vi "Measurement.vi"(0 "Position":T3(array[cluster]) {"Z" format="%.1f"; "Y" format="%.1f"; "X" format="%.1f"}, 1 "setup":T4=enum."Show Setup", 2 "Post Process":T2, 4 "File":T5, 5 "Results file":path, 7 "Raw data file":path, 11 "Setup filename":string) -> (14 "2nd plot":cluster{"X array":dbl[], "Y array":dbl[]}[](graph), 19 "Status Out":T1)   [LabVIEW 2015]
uses:
  Anemometry Sub Vis/Controls/Save_Data.ctl
  Anemometry Sub Vis/Controls/Setup.ctl
  Anemometry Sub Vis/Controls/Graph_Type.ctl
  Anemometry Sub Vis/Controls/Post_Process.ctl
  Anemometry Sub Vis/Gen Trav/Multi_Run_Status.ctl
  Anemometry Sub Vis/Controls/Inst_type.ctl
  ADAM Client/Sub VIs/ADAM Controls/Traverse_Level_State.ctl
  Anemometry Sub Vis/File/Setup_Filetype.ctl
  Anemometry Sub Vis/Globals/Meas_global.vi
  Anemometry Sub Vis/Globals/Trav_pos_global.vi
  Anemometry Sub Vis/Globals/Plug_in_data_global.vi
  Anemometry Sub Vis/Globals/Dynamic_call_global.ph.vi
  Anemometry Sub Vis/Globals/Preference_global.vi
  Anemometry Sub Vis/Globals/Constants_global.vi
  Anemometry Sub Vis/Globals/Extra_Commands_Global.vi
  Anemometry Sub Vis/Globals/LDA_meas_global_2.vi
  Anemometry Sub Vis/Globals/LDA_meas_global_1.vi
  Anemometry Sub Vis/Acquisition/PWA/PWAtasksGLOBAL.vi
  Anemometry Sub Vis/Acquisition/Data_Translation/DataTranslation_global.vi
  Anemometry Sub Vis/Globals/Gas_management_global.vi
panel:
  in  "PP next block":bool
  out "Pause message":string
  out "Statistics":string[][](table)
  out "Actual Sampling freq":dbl=100.0 format="%.1f"
  in  "Desired Sampling freq (Hz)":dbl=100.0 format="%.1f"
  out "Current Block No":i32=5 caption="Current Block"
  in  "Pause":bool
  in  "No of Blocks":i32=5
  in  "stop":bool
  in  "No of samples":i32=1000 min=0 step=1
  in  "Tab Control":T6(tab)
  in  "Second Graph":T8={"Plot 1"=2, "Plot 2"=1, "Save graph"=0, "Plot Type"=enum."Vel histogram"} {"Save graph" items=["Do not save plot", "Save plot"]; "Plot 2" items=["Nothing", "V"]; "Plot 1" items=["Nothing", "V"]}
  in  "First Graph":T8={"Plot 1"=1, "Plot 2"=2, "Save graph"=0, "Plot Type"=enum."Velocity trace"} {"Save graph" items=["Do not save plot", "Save plot"]; "Plot 2" items=["Nothing", "V"]; "Plot 1" items=["Nothing", "V"]}
  out "First plot":cluster{"X array":dbl[], "Y array":dbl[]}[](graph)
  in  "Comments":string
  out "uv":dbl[][](graph)=[[-0.041806189081711534, -0.046435429052714985, -0.04035660097427599, -0.042187605126076694, -0.042052555599004206]]
  out "u^4":dbl[][](graph)
  out "u^3":dbl[][](graph)
  out "u^2":dbl[][](graph)=[[0.09743628875280319, 0.10575821456272283, 0.10126262927293661, 0.09890442087602569, 0.1022948212436432]]
  out "U":dbl[][](graph)=[[0.8295029456391334, 0.8915896983798417, 0.8415763502225625, 0.8394746126219594, 0.8466062785395404]]
  in  "Block average display control":cluster{"Name":string, "Include":bool}[](array[cluster])=[{"Name"="FF (C)", "Include"=FALSE}]
  in  "No of bins in histogram":i32=100
  out "Measurement time (min)":dbl=6.0 format="%.2f"
  in  "Correlate?":T9(ring)
  out "Diagnostic info":string[][](table)
  out "Array U":dbl[][](array[numeric]) format="%.2e"
  out "Array u^2":dbl[][](array[numeric]) format="%.2e"
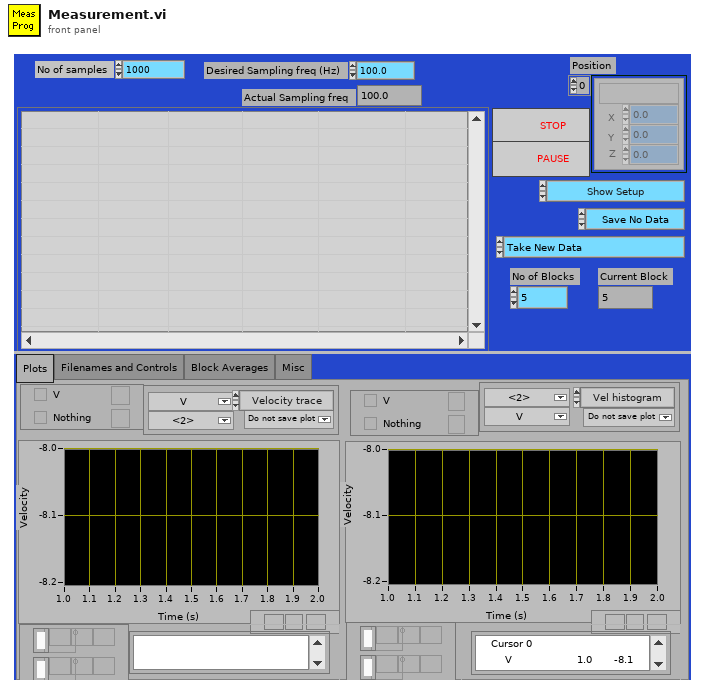
[diagram p1: front panel]
types:
  T1 = typedef "Multi_Run_Status.ctl" = enum16{"Continue", "Jump to Next Point", "Jump to Next Row", "Jump To Fall Back", "Terminate Run"}
  T2 = typedef "Post_Process.ctl" = enum16{"Take New Data", "Post Process Raw Data File"}
  T3 = cluster{"Name":string, "X":dbl, "Y":dbl, "Z":dbl}[]
  T4 = typedef "Setup.ctl" = enum16{"Run Program", "Show Setup", "Save Current Setup", "Setup Front Panel"}
  T5 = typedef "Save_Data.ctl" = enum16{"Save No Data", "Save Data"}
  T6 = enum32{"Plots", "Filenames and Controls", "Block Averages", "Misc"}
  T7 = typedef "Graph_Type.ctl" = enum16{"Show no graph", "Voltage trace", "Velocity trace", "Vel histogram", "Spectrum", "f.E(f) v Log f", "Auto-Corr"}
  T8 = cluster{"Plot 1":u16, "Plot 2":u16, "Save graph":u16, "Plot Type":T7}
  T9 = enum16{"Cross correlation off", "Show correlation panel", "Correlate without activating panel"}
  T10 = enum32{"Bad", "Idle", "Run top level", "Running"}
  T11 = cluster{"Name":string, "X":dbl, "Y":dbl, "Z":dbl}
  T12 = enum16{"Velocity", "Transit time", "Arrival time"}
  T13 = enum16{"Save no data", "Save data in new files", "Save data in existing files"}
  T14 = typedef "Inst_type.ctl" = enum16{"Propeller anemometer", "Raw voltage", "Pressure Transducer", "Pitot-static tube", "Preston tube", "Hot wire", "Cross wire 1", "Cross wire 2", "Generic Linear", "Generic Polynomial", "Generic BackPoly", "Fast FID", "Thermocouple", "Cold wire", "Pulsed Wire", "LDA Vel", "LDA Tran time", "LDA Arr time", "Microphone"}
  T15 = enum16{"Zero or one", "One", "Zero or more", "One or more"}
  T16 = cluster{"Weighting":dbl[], "Time (ms)":dbl[], "Voltage":dbl[], "Eng Values":dbl[]}
  T17 = typedef "Traverse_Level_State.ctl" = enum16{"Running", "Complete"}
  T18 = typedef "Setup_Filetype.ctl" = enum16{"Measurement Setups", "Calibration Setups", "General", "Results File Plotter Setups", "Speed Calib Tweaks"}
  T19 = typedef "Traverse_cluster.ctl" = cluster{"Start X":sgl, "Start Y":sgl, "Start Z":sgl, "End X":sgl, "End Y":sgl, "End Z":sgl, "No. of pts.":i32, "Spacing":T20, "Filename":path, "Tunnel Speed":dbl, "Averaging time (min)":dbl, "Extra Commands":string, "Carrier_1 Q (l/min)":dbl, "Carrier_2 Q (l/min)":dbl, "Trace Gas Concentration (%)":dbl, "Specific Arguments":string, "Comments":string, "Row No":i32, "Row Type Selector":T21, "Completion time":string, "Row Duration (mins)":dbl, "No. of Valid pts.":i32, "Meas Setup File":string}
  T20 = typedef "Spacing.ctl" = enum16{"Linear", "Log", "Gauss", "Specified", "N/A"}
  T21 = typedef "Multi_run_mode.ctl" = enum16{"Move Traverse Only", "Set Tunnel Speed Only", "Set Source Only", "Set Measurement Conditions", "Single Measurement", "Vertical Profile", "Lateral Profile", "Longitudinal Profile", "Explore Volume", "Multi-Axis Profile", "Auto Calibrate", "Meas Fast FID Bkgnd", "Check Beam Power", "Scanning Valve Measurement", "Run VI Named:", "Set ADAM Ch", "Wait (minutes)", "Send Message", "Synchronize With:", "Fall Back to this Row", "Turn Off Row Repeating", "Blank Row", "Traverse 3D Volume"}
  T22 = typedef "Analysis_info_cluster.ctl" = cluster{"Colour":u32, "Inst type":T14, "Inst name":string, "Symbol":string, "Code name":string, "Extra Info":string, "Inst Array":T23, "Extra Titles":string[], "Extra Values":string[], "U":dbl, "u^2":dbl, "u^3":dbl, "u^4":dbl, "Skew_u":dbl, "Kurt_u":dbl, "Sd Error in Mean":dbl, "% u'/U":dbl, "X":dbl, "Y":dbl, "Z":dbl, "Timescale integral to 25%":dbl, "Sd Error in Variance":dbl, "Calib File":path, "Calib Constants":dbl[], "Output Position":bool, "Full Stats":bool, "Av Sampling Rate":dbl, "Av No of Samples":dbl, "Total Meas Time (s)":dbl, "ADAM Ch Name":string}
  T23 = typedef "Instrument_Array.ctl" = enum16{"PWA", "LDA", "Analogue"}
  T24 = typedef "LDA_Setup.ctl" = cluster{"dimensions":enum16{"1D", "2D"}, "Analogue Freq Multiplier":dbl}
  T25 = enum16{"Velocity", "Transit time", "Arrival time"}[]
  T26 = typedef "BSA_Type.ctl" = enum16{"57N11", "BSA F60"}
  T27 = typedef "BSA_info_Cluster.ctl" = cluster{"GPIB Address":string, "No of Check Bytes":i32, "Extra Info":string, "COLOUR":u32, "Wavelength (nm)":dbl}
  T28 = typedef "Ch_and_Spans.ctl" = cluster{"high limit (10V)":sgl, "low limit (-10V)":sgl, "Ch No":i16, "Var name":string, "Use Latest Calib":bool}
  T29 = cluster{"Weighting":dbl[], "Time (ms)":dbl[], "Voltage":dbl[], "Eng Values":dbl[]}[]
  T30 = cluster{"Insts for plotting[0]":u16, "Insts for plotting[1]":u16}
  T31 = typedef "PWA_Data.ctl" = enum16{"No PWA Data", "One Ch PWA"}
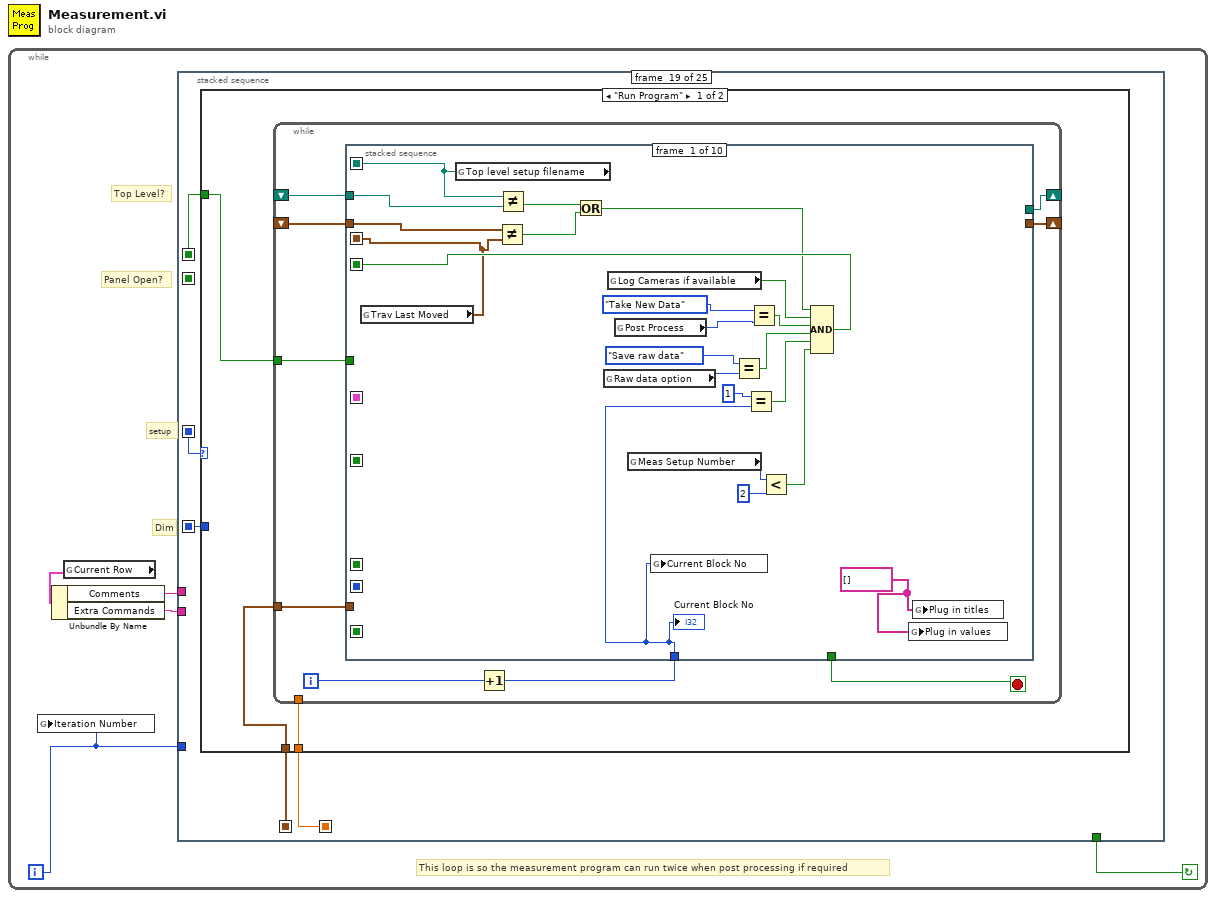
[diagram p0: block diagram]
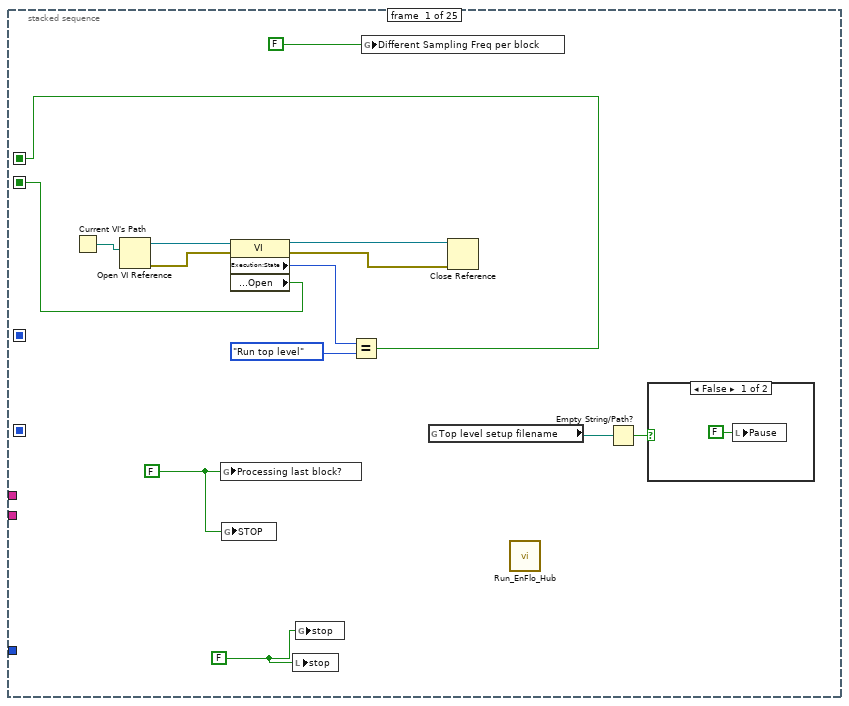
[diagram p2: hidden frame]
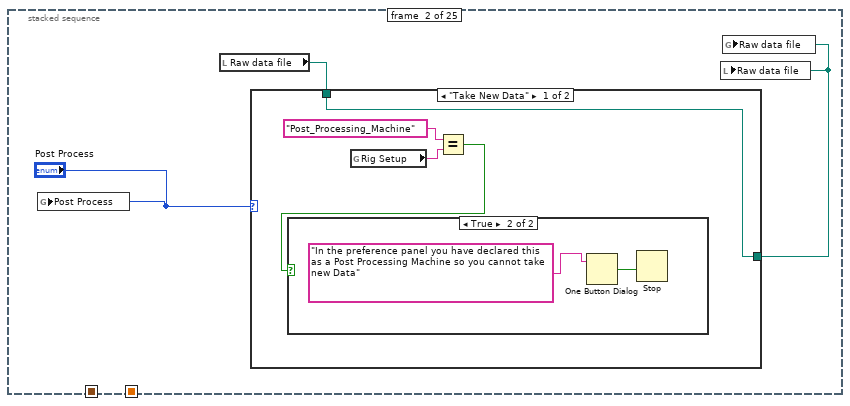
[diagram p4: hidden frame]
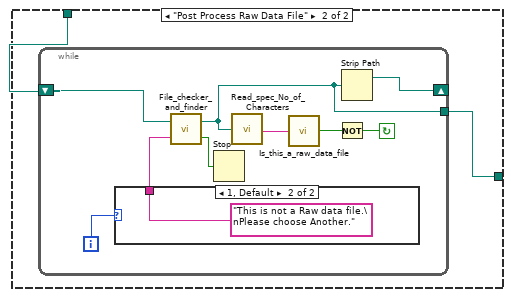
[diagram p6: hidden frame]
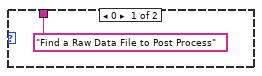
[diagram p7: hidden frame]
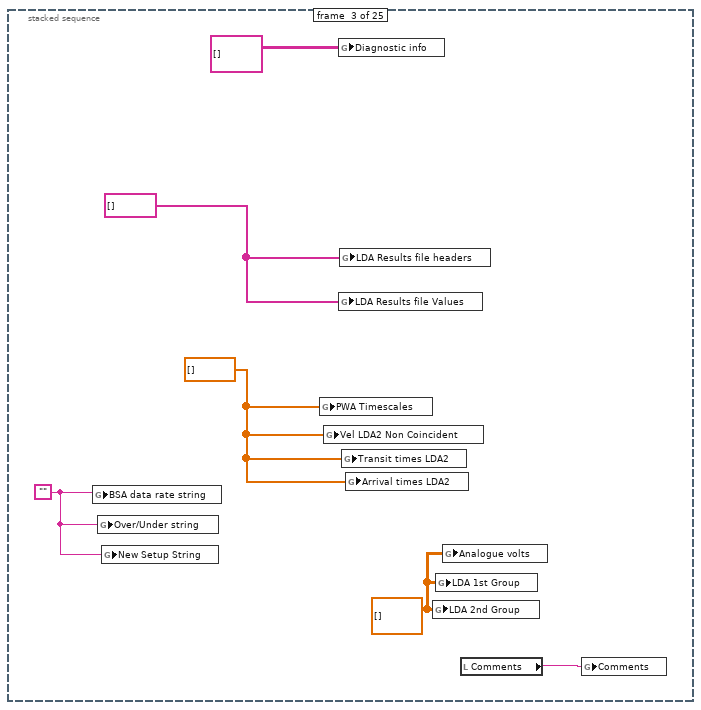
[diagram p8: hidden frame]
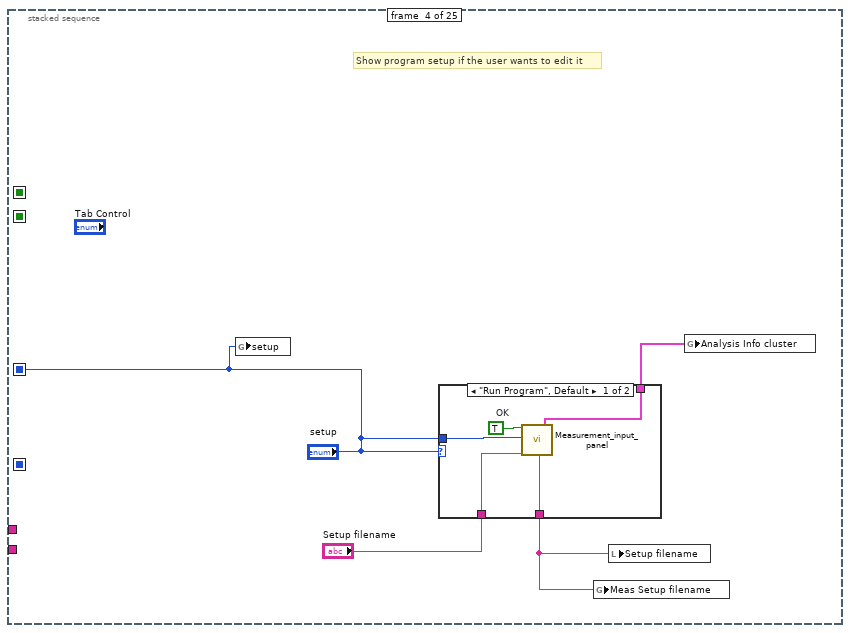
[diagram p9: hidden frame]
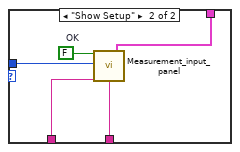
[diagram p10: hidden frame]
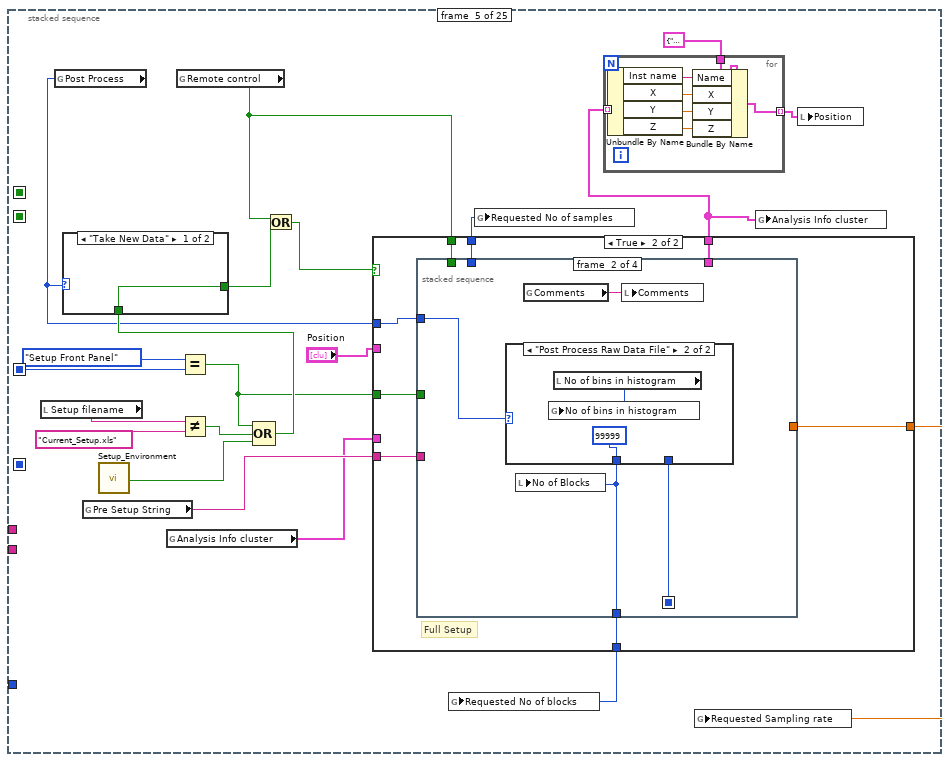
[diagram p11: hidden frame]
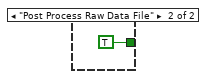
[diagram p12: hidden frame]
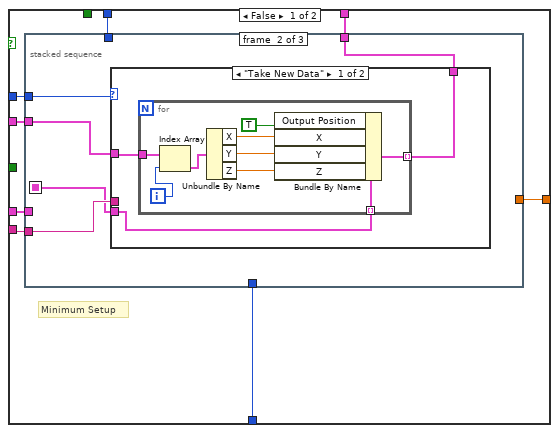
[diagram p13: hidden frame]
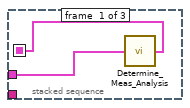
[diagram p14: hidden frame]
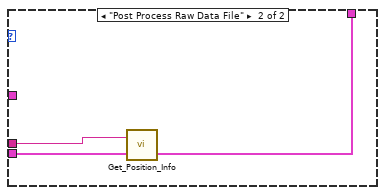
[diagram p15: hidden frame]
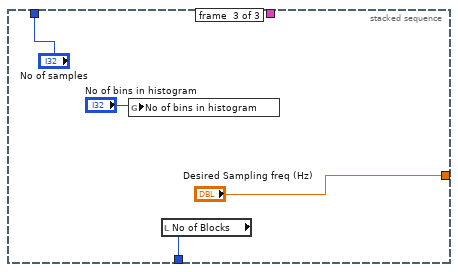
[diagram p16: hidden frame]
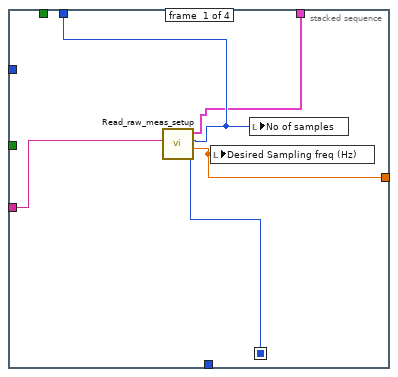
[diagram p17: hidden frame]
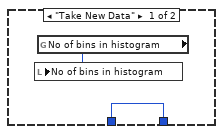
[diagram p18: hidden frame]
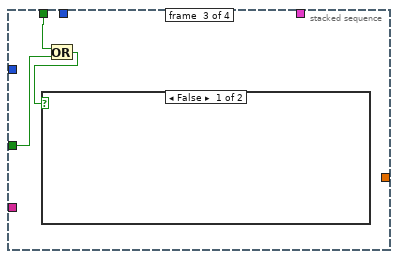
[diagram p19: hidden frame]
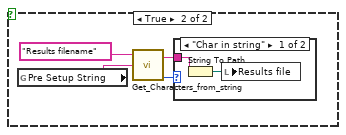
[diagram p20: hidden frame]
diagram:
  n1 = while {
    i -> [w2]
    stop <- w3 continue-if-true
    # "This loop is so the measurement program can run twice when post processing if required"
    # "Panel Open?"
    # "Top Level?"
    # "setup"
    # "Dim"
    n2 = global write "Meas_global.vi" "Iteration Number"(w2) -> ()
    n3 = global read "Trav_pos_global.vi" "Current Row"() -> (w4:T19)
    n4 = Unbundle By Name(w4) -> ("Comments"=w5:string, "Extra Commands"=w1:string)
    n5 = stacked-sequence {
      seq-local: [_ _ _ _ _ _ _ _ w215 _ _ _ _ _ _ _ _ _ _ _ _ _ _ _ _] -> [_ _ _ _ _ _ _ _ _ _ _ _ _ _ _ _ _ _ w843 _ _ _ _ _ _]
      seq-local: [_ _ _ "setup" _ _ _ _ _ _ _ _ _ _ _ _ _ _ _ _ _ _ _ _ _] -> [_ _ _ _ w75 _ w179 _ w214 w303 _ _ _ _ w725 w744 w751 _ w844 w1106 w1157 w1238 _ _ w1359]
      seq-local: [_ _ _ _ _ _ _ _ _ _ _ _ _ _ _ _ w748 _ _ _ _ _ _ _ _] -> [_ _ _ _ _ _ _ _ _ _ _ _ _ _ _ _ _ _ w842 w1096 _ _ _ _ _]
      seq-local: [w10 _ _ _ _ _ _ _ _ _ _ _ _ _ _ _ _ _ _ _ _ _ _ _ _] -> [_ _ _ _ _ _ _ _ _ w283 _ _ _ _ w722 _ _ _ w841 _ _ _ _ _ _]
      seq-local: [w9 _ _ _ _ _ _ _ _ _ _ _ _ _ _ _ _ _ _ _ _ _ _ _ _] -> [_ _ _ _ _ _ _ _ _ _ _ _ w516 _ _ _ _ _ _ _ _ _ _ _ _]
      seq-local: [_ _ _ _ _ _ _ _ _ _ _ _ _ _ _ _ w746 _ _ _ _ _ _ _ _] -> [_ _ _ _ _ _ _ _ _ _ _ _ _ _ _ _ _ _ w840 _ _ _ _ _ _]
      tunnel: w5 -> [_ _ _ _ _ _ _ w212 _ _ _ _ _ _ _ _ _ _ _ _ _ _ _ w1328 _]
      tunnel: w2 -> [_ _ _ _ _ _ _ _ _ _ _ _ _ _ _ _ _ _ _ _ _ _ _ w1323 _]
      tunnel: [_ _ _ _ _ _ _ _ _ _ _ _ _ _ _ _ _ _ _ _ _ _ _ w1322 _] -> w3
      tunnel: w1 -> [_ _ _ _ _ _ _ _ _ _ _ _ _ _ _ _ _ _ _ _ w1156 _ _ _ _]
      frame #0 {
        w18 = FALSE ("Processing last block?")
        w19 = FALSE ("stop")
        n6 = Current VI's Path() -> (path=w11:path)
        n7 = Open VI Reference(vi path=w11) -> (vi reference=w12:refnum<vi>, error out=w13:errorcluster)  [unwired: 1 in, 4 out]
        n8 = global write "Meas_global.vi" "Processing last block?"(w18) -> ()
        n9 = global write "PWAtasksGLOBAL.vi" "STOP"(w18) -> ()
        n10 = property class="VI"(reference=w12, error in=w13) -> (reference out=w14:refnum<vi>, error out=w15:errorcluster, "Execution:State"=w16:T10, "Front Panel.Open"=w9:bool)
        n11 = local write "stop"(w19) -> ()
        n12 = global write "Meas_global.vi" "stop"(w19) -> ()
        n13 = Equal?(x=w16, y=T10."Run top level" ("Exec.State")) -> (x = y?=w10:bool)
        n14 = global write "DataTranslation_global.vi" "Different Sampling Freq per block"(FALSE ("Different Sampling Freq per block")) -> ()
        n15 = global read "Trav_pos_global.vi" "Top level setup filename"() -> (w7:path)
        n16 = Close Reference(reference=w14, error in (no error)=w15) -> ()  [unwired: 1 out]
        n17 = call "Run_EnFlo_Hub.vi"() -> ()  [unwired: 8 out]
        n18 = Empty String/Path?(string/path=w7) -> (empty?=w6:bool)
        n19 = case shown="False" w6 {
          frame False {
            n20 = local write "Pause"(FALSE ("Pause")) -> ()
          }
          frame True {
          }
        }
      }
      frame #1 {
        n21 = global write "Meas_global.vi" "Post Process"("Post Process") -> ()
        n22 = local read "Raw data file"() -> (w23:path)
        n23 = case shown="\"Take New Data\"" "Post Process" {
          tunnel: [w27 w31] -> w22
          tunnel: w23 -> [w27 w30]
          frame "Take New Data" {
            n24 = global read "Preference_global.vi" "Rig Setup"() -> (w26:string)
            n25 = Equal?(x="Post_Processing_Machine" ("Rig Setup"), y=w26) -> (x = y?=w24:bool)
            n26 = case shown="True" w24 {
              frame False {
              }
              frame True {
                n27 = One Button Dialog(message="In the preference panel you have declared this as a Post Processing Machine so you cannot take new Data") -> (true=w28:bool)  [unwired: 1 in]
                n28 = Stop(stop? (T)=w28) -> ()
              }
            }
          }
          frame "Post Process Raw Data File" {
            n29 = while {
              tunnel: [w33] -> w31
              shift-left: w30 -> [w35]
              shift-right: [w34] -> _
              i -> [w36]
              stop <- w37 continue-if-true
              n30 = case shown="1, Default" w36 {
                tunnel: ["Find a Raw Data File to Post Process" ("Promp if not found") "This is not a Raw data file.\nPlease choose Another." ("Promp if not found")] -> w40
                frame 0 {
                }
                frame 1, Default {
                }
              }
              n31 = call "File_checker_and_finder.vi"("Promp if not found"=w40, "Filename In"=w35) -> ("cancelled"=w32:bool, "Filename Out"=w33:path)
              n32 = Stop(stop? (T)=w32) -> ()
              n33 = call "Read_spec_No_of_Characters.vi"("Filename"=w33) -> ("character string"=w39:string)  [unwired: 1 out]
              n34 = call "Is_this_a_raw_data_file.vi"("character string"=w39) -> ("Raw Dat File?"=w38:bool)  [unwired: 2 out]
              n35 = Not(x=w38) -> (.not. x?=w37:bool)
              n36 = Strip Path(path=w33) -> (stripped path=w34:path)  [unwired: 1 out]
            }
          }
        }
        n37 = local write "Raw data file"(w22) -> ()
        n38 = global write "Meas_global.vi" "Raw data file"(w22) -> ()
      }
      frame #2 {
        w43 = dbl[][] [] ("LDA 2nd Group")
        w44 = dbl[] [] ("LDA Timescales")
        w46 = string[] [] ("Plug in values")
        w48 = ""
        n39 = global write "Meas_global.vi" "BSA data rate string"(w48) -> ()
        n40 = global write "Meas_global.vi" "Over/Under string"(w48) -> ()
        n41 = global write "Meas_global.vi" "New Setup String"(w48) -> ()
        n42 = global write "PWAtasksGLOBAL.vi" "PWA Timescales"(w44) -> ()
        n43 = global write "LDA_meas_global_2.vi" "Vel LDA2 Non Coincident"(w44) -> ()
        n44 = global write "Meas_global.vi" "Diagnostic info"(string[][] [] ("Diagnostic info")) -> ()
        n45 = global write "LDA_meas_global_1.vi" "LDA Results file Values"(w46) -> ()
        n46 = global write "LDA_meas_global_1.vi" "LDA Results file headers"(w46) -> ()
        n47 = global write "LDA_meas_global_2.vi" "Transit times LDA2"(w44) -> ()
        n48 = global write "LDA_meas_global_2.vi" "Arrival times LDA2"(w44) -> ()
        n49 = global write "LDA_meas_global_2.vi" "LDA 2nd Group"(w43) -> ()
        n50 = global write "LDA_meas_global_2.vi" "LDA 1st Group"(w43) -> ()
        n51 = global write "Meas_global.vi" "Analogue volts"(w43) -> ()
        n52 = local read "Comments"() -> (w47:string)
        n53 = global write "Meas_global.vi" "Comments"(w47) -> ()
      }
      frame #3 {
        # "Show program setup if the user wants to edit it"
        n54 = global write "Meas_global.vi" "setup"("setup") -> ()
        n55 = case shown="\"Run Program\", Default" "setup" {
          tunnel: [w56 w61] -> w52
          tunnel: "Setup filename" -> [w55 w60]
          tunnel: [w54 w59] -> w50
          tunnel: "setup" -> [w53 w58]
          frame "Run Program", Default {
            w57 = TRUE  # OK
            n56 = call "Measurement_input_panel.vi"("OK"=w57, "setup"=w53, "Setup filename"=w55) -> ("Setup filename out"=w54:string, "Analysis Info cluster"=w56:T22[])  [unwired: 15 out]
          }
          frame "Show Setup" {
            w62 = FALSE  # OK
            n57 = call "Measurement_input_panel.vi"("OK"=w62, "setup"=w58, "Setup filename"=w60) -> ("Setup filename out"=w59:string, "Analysis Info cluster"=w61:T22[])  [unwired: 15 out]
          }
        }
        n58 = global write "Meas_global.vi" "Meas Setup filename"(w50) -> ()
        n59 = local write "Setup filename"(w50) -> ()
        n60 = global write "Meas_global.vi" "Analysis Info cluster"(w52) -> ()
      }
      frame #4 {
        n61 = local read "Setup filename"() -> (w79:string)
        n62 = global read "Meas_global.vi" "Post Process"() -> (w74:T2)
        n63 = global read "Meas_global.vi" "Pre Setup String"() -> (w70:string)
        n64 = call "Setup_Environment.vi"() -> ("First Time"=w71:bool)  [unwired: 1 in]
        n65 = global read "Meas_global.vi" "Analysis Info cluster"() -> (w67:T22[])
        n66 = global read "Meas_global.vi" "Remote control"() -> (w69:bool)
        n67 = Equal?(x=Setup."Setup Front Panel" ("setup"), y=w75) -> (x = y?=w68:bool)
        n68 = Not Equal?(x=w79, y="Current_Setup.xls" ("Setup filename")) -> (x != y?=w77:bool)
        n69 = Compound Arithmetic op=OR(w68, w77, w71) -> (w76:bool)
        n70 = case shown="\"Take New Data\"" w74 {
          tunnel: [w91 TRUE] -> w83
          tunnel: w76 -> [w91 _]
          frame "Take New Data" {
          }
          frame "Post Process Raw Data File" {
          }
        }
        n71 = Or(x=w69, y=w83) -> (x .or. y?=w82:bool)
        n72 = case shown="True" w82 {
          tunnel: w74 -> [w96 w134]
          tunnel: [w100 w133] -> w72
          tunnel: [w99 w128] -> w81
          tunnel: [w98 w132] -> w80
          tunnel: [w97 w131] -> w66
          tunnel: w70 -> [w95 w130]
          tunnel: "Position" -> [w94 _]
          tunnel: w69 -> [_ w129]
          tunnel: w68 -> [_ w127]
          tunnel: w67 -> [w93 _]
          frame False {
            # "Minimum Setup"
            n73 = stacked-sequence {
              seq-local: [w101 _ _] -> [_ w103 _]
              tunnel: [_ _ "Desired Sampling freq (Hz)"] -> w100
              tunnel: [_ _ w125] -> w99
              tunnel: [_ _ "No of samples"] -> w98
              tunnel: [_ w106 _] -> w97
              tunnel: w96 -> [_ w107 _]
              tunnel: w95 -> [_ w105 _]
              tunnel: w94 -> [_ w104 _]
              tunnel: w93 -> [w102 _ _]
              frame #0 {
                n74 = call "Determine_Meas_Analysis.vi"("Analysis info Cluster In"=w102) -> ("Analysis info Cluster Out"=w101:T22[])
              }
              frame #1 {
                n75 = case shown="\"Take New Data\"" w107 {
                  tunnel: [w108 w120] -> w106
                  tunnel: w104 -> [w110 _]
                  tunnel: w105 -> [_ w121]
                  tunnel: w103 -> [w109 w122]
                  frame "Take New Data" {
                    n76 = for {
                      tunnel: w110 -> [w113]
                      tunnel: w109 -> [w119] mode=indexing
                      tunnel: [w115] -> w108 mode=indexing
                      i -> [w114]
                      n77 = Index Array(array=w113, index=w114) -> (element=w112:T11)
                      n78 = Unbundle By Name(w112) -> ("X"=w116:dbl, "Y"=w117:dbl, "Z"=w118:dbl)
                      n79 = Bundle By Name(cluster=w119, "Output Position"=TRUE, "X"=w116, "Y"=w117, "Z"=w118) -> (w115:T22)
                    }
                  }
                  frame "Post Process Raw Data File" {
                    n80 = call "Get_Position_Info.vi"("Analysis Info cluster"=w122, "Setup file string"=w121) -> ("Analysis Info cluster 2"=w120:T22[])  [unwired: 1 in]
                  }
                }
              }
              frame #2 {
                n81 = global write "Meas_global.vi" "No of bins in histogram"("No of bins in histogram") -> ()
                n82 = local read "No of Blocks"() -> (w125:i32)
              }
            }
          }
          frame True {
            # "Full Setup"
            n83 = stacked-sequence {
              seq-local: [w136 _ _ _] -> [_ w141 _ _]
              tunnel: w134 -> [_ w142 _ w157]
              tunnel: [w139 _ _ _] -> w133
              tunnel: [w138 _ _ _] -> w132
              tunnel: [w135 _ _ _] -> w131
              tunnel: w130 -> [w137 _ _ _]
              tunnel: w129 -> [_ _ w150 _]
              tunnel: [_ w140 _ _] -> w128
              tunnel: w127 -> [_ _ w149 _]
              frame #0 {
                n84 = call "Read_raw_meas_setup.vi"("Setup file string"=w137) -> ("No of Blocks"=w136:i32, "Sampling freq (Hz)"=w139:dbl, "No of samples"=w138:i32, "Analysis Info cluster 2"=w135:T22[])  [unwired: 5 out]
                n85 = local write "Desired Sampling freq (Hz)"(w139) -> ()
                n86 = local write "No of samples"(w138) -> ()
              }
              frame #1 {
                n87 = case shown="\"Post Process Raw Data File\"" w142 {
                  tunnel: [w145 99999 ("No of Blocks")] -> w140
                  tunnel: w141 -> [w145 _]
                  frame "Take New Data" {
                    n88 = global read "Meas_global.vi" "No of bins in histogram"() -> (w144:i32)
                    n89 = local write "No of bins in histogram"(w144) -> ()
                  }
                  frame "Post Process Raw Data File" {
                    n90 = local read "No of bins in histogram"() -> (w146:i32)
                    n91 = global write "Meas_global.vi" "No of bins in histogram"(w146) -> ()
                  }
                }
                n92 = local write "No of Blocks"(w140) -> ()
                n93 = global read "Meas_global.vi" "Comments"() -> (w143:string)
                n94 = local write "Comments"(w143) -> ()
              }
              frame #2 {
                n95 = Or(x=w150, y=w149) -> (x .or. y?=w148:bool)
                n96 = case shown="False" w148 {
                  frame False {
                  }
                  frame True {
                    n97 = global read "Meas_global.vi" "Pre Setup String"() -> (w151:string)
                    n98 = call "Get_Characters_from_string.vi"("Input string"=w151, "Variable name"="Results filename") -> ("Status"=w154:enum16{"Char in string", "Char not in string"}, "Value"=w153:string)  [unwired: 1 in]
                    n99 = case shown="\"Char in string\"" w154 {
                      tunnel: w153 -> [w156 _]
                      frame "Char in string" {
                        n100 = String To Path(string=w156) -> (path=w155:path)
                        n101 = local write "Results file"(w155) -> ()
                      }
                      frame "Char not in string" {
                      }
                    }
                  }
                }
              }
              frame #3 {
                n102 = case shown="\"Post Process Raw Data File\"" w157 {
                  frame "Take New Data" {
                    n103 = global read "Meas_global.vi" "Second Graph"() -> (w158:T8)
                    n104 = global read "Meas_global.vi" "First Graph"() -> (w159:T8)
                    n105 = local write "Second Graph"(w158) -> ()
                    n106 = local write "First Graph"(w159) -> ()
                  }
                  frame "Post Process Raw Data File" {
                  }
                }
              }
            }
          }
        }
        n107 = global write "Meas_global.vi" "Requested No of blocks"(w81) -> ()
        n108 = global write "Meas_global.vi" "Requested No of samples"(w80) -> ()
        n109 = for {
          tunnel: w66 -> [w90] mode=indexing
          tunnel: [w86] -> w64 mode=indexing
          tunnel: T11 {"Name"="", "X"=0.0, "Y"=0.0, "Z"=0.0} ("Position") -> [w85]
          n110 = Unbundle By Name(w90) -> ("Inst name"=w84:string, "X"=w87:dbl, "Y"=w88:dbl, "Z"=w89:dbl)
          n111 = Bundle By Name(cluster=w85, "Name"=w84, "X"=w87, "Y"=w88, "Z"=w89) -> (w86:T11)
        }
        n112 = global write "Meas_global.vi" "Requested Sampling rate"(w72) -> ()
        n113 = global write "Meas_global.vi" "Analysis Info cluster"(w66) -> ()
        n114 = local write "Position"(w64) -> ()
      }
      frame #5 {
        n115 = global read "Meas_global.vi" "Post Process"() -> (w160:T2)
        n116 = case shown="\"Post Process Raw Data File\"" w160 {
          tunnel: [w163 w164] -> w161
          frame "Take New Data" {
            n117 = Get Date/Time In Seconds() -> (seconds since 1Jan1904=w162:timestamp)
            n118 = To Double Precision Float(number=w162) -> (double precision float=w163:dbl)
          }
          frame "Post Process Raw Data File" {
            n119 = global read "Meas_global.vi" "Pre Setup String"() -> (w167:string)
            n120 = call "Get_Characters_from_string.vi"("Input string"=w167, "Variable name"="Seconds since 1/1/04") -> ("Value"=w165:string)  [unwired: 1 in, 1 out]
            n121 = call "String_2_Number.vi"("Value"=w165) -> ("Numeric"=w164:dbl)
          }
        }
        n122 = global write "Meas_global.vi" "Time Data was Aquired"(w161) -> ()
      }
      frame #6 {
        n123 = global read "Dynamic_call_global.ph.vi" "Initial Plug Ins"() -> (w184:string[])
        n124 = global read "Trav_pos_global.vi" "Source Control?"() -> (w181:bool)
        n125 = local read "Setup filename"() -> (w172:string)
        n126 = global read "Meas_global.vi" "Post Process"() -> (w170:T2)
        n127 = Search 1D Array(1D array=w184, element="Puff_using_Arduino.vi") -> (index of element=w182:i32)  [unwired: 1 in]
        n128 = Equal?(x=w170, y=Post_Process."Take New Data" ("Post Process")) -> (x = y?=w168:bool)
        n129 = Equal?(x=Setup."Run Program" ("setup"), y=w179) -> (x = y?=w177:bool)
        n130 = Less Than 0?(x=w182) -> (x < 0?=w174:bool)
        n131 = Not Equal?(x=w172, y="Meas_FF_Bkgnd_Setup.xls") -> (x != y?=w176:bool)
        n132 = Not Equal?(x=w172, y="Auto_Calib_Setup.xls") -> (x != y?=w171:bool)
        n133 = Compound Arithmetic op=AND(w181, w177, w176, w171, w168) -> (w175:bool)
        n134 = case shown="True" w175 {
          tunnel: w174 -> [_ w185]
          frame False {
          }
          frame True {
            n135 = global read "Gas_management_global.vi" "Source Live"() -> (w186:bool)
            n136 = Not(x=w186) -> (.not. x?=w187:bool)
            n137 = Select(t=w186, s=w185, f=w187) -> (s? t:f=w188:bool)
            n138 = global read "Preference_global.vi" "Default Source Establishment Time (s)"() -> (w189:dbl)
            n139 = case shown="False" w188 {
              tunnel: w189 -> [w191 w204]
              tunnel: w185 -> [w190 _]
              frame False {
                n140 = stacked-sequence {
                  tunnel: w191 -> [_ w200]
                  tunnel: w190 -> [w192 _]
                  frame #0 {
                    n141 = case shown="False" w192 {
                      tunnel: [w197 w199] -> w194
                      tunnel: [w196 w198] -> w193
                      frame True {
                        w196 = u32 0  # Time to hold source OFF (microseconds)
                        w197 = u32 1  # Time to hold source ON (microseconds)
                      }
                      frame False {
                        w198 = u32 1  # Time to hold source OFF (microseconds)
                        w199 = u32 0  # Time to hold source ON (microseconds)
                      }
                    }
                    n142 = call "Arduino_Timed_Release.vi"("Time to hold source ON (microseconds)"=w194, "Time to hold source OFF (microseconds)"=w193, "Number of cycles"=u16 1) -> ()  [unwired: 2 out]
                  }
                  frame #1 {
                    n143 = Greater Than 0?(x=w200) -> (x > 0?=w201:bool)
                    n144 = case shown="True" w201 {
                      tunnel: w200 -> [_ w202]
                      frame False {
                      }
                      frame True {
                        n145 = call "Wait_Seconds_with_display.vi"("Message"="Est Source", "Seconds to wait"=w202) -> ()  [unwired: 2 out]
                      }
                    }
                  }
                }
              }
              frame True {
                n146 = global read "Gas_management_global.vi" "Source Live Last changed"() -> (w208:timestamp)
                n147 = Get Date/Time In Seconds() -> (seconds since 1Jan1904=w209:timestamp)
                n148 = Subtract(x=w209, y=w208) -> (x-y=w207:dbl)
                n149 = Subtract(x=w204, y=w207) -> (x-y=w205:dbl)
                n150 = call "Wait_Seconds_with_display.vi"("Message"="Est Source", "Seconds to wait"=w205) -> ()  [unwired: 2 out]
              }
            }
          }
        }
      }
      frame #7 {
        n151 = local read "Comments"() -> (w213:string)
        n152 = Concatenate Strings(w212, w213) -> (w211:string)
        n153 = call "Text_without_format.vi"("Input string"=w211) -> ("Output string"=w210:string)
        n154 = local write "Comments"(w210) -> ()
        n155 = global write "Meas_global.vi" "Comments"(w210) -> ()
      }
      frame #8 {
        n156 = global read "Meas_global.vi" "LDA set up"() -> (w216:T24)
        n157 = Unbundle By Name(w216) -> ("dimensions"=w215:enum16{"1D", "2D"})
        n158 = global read "Meas_global.vi" "LDA data"() -> (w223:enum16{"No LDA data", "Take LDA data"})
        n159 = global read "Meas_global.vi" "Post Process"() -> (w225:T2)
        n160 = Equal?(x=w214, y=Setup."Show Setup" ("setup")) -> (x = y?=w217:bool)
        n161 = Equal?(x=w223, y=enum16{"No LDA data", "Take LDA data"}."Take LDA data" ("LDA data")) -> (x = y?=w219:bool)
        n162 = Equal?(x=w225, y=Post_Process."Take New Data" ("Post Process")) -> (x = y?=w220:bool)
        n163 = Compound Arithmetic op=AND(w219, w220) -> (w218:bool)
        n164 = case shown="True" w218 {
          tunnel: w215 -> [_ w234]
          tunnel: w214 -> [_ w233]
          tunnel: w217 -> [_ w231]
          frame False {
            n165 = Build Array(T12."Velocity", T12."Transit time", T12."Arrival time") -> (w226:T25)
            n166 = global write "LDA_meas_global_1.vi" "Number of measured quantities"(3 ("Number of measured quantities")) -> ()
            n167 = global write "LDA_meas_global_2.vi" "data type"(w226) -> ()
            n168 = global write "LDA_meas_global_1.vi" "data type"(w226) -> ()
          }
          frame True {
            n169 = global read "LDA_meas_global_1.vi" "BSA Type"() -> (w232:T26)
            n170 = case shown="\"BSA F60\"" w232 {
              tunnel: w234 -> [w236 _]
              tunnel: w233 -> [w235 _]
              tunnel: w231 -> [_ w272]
              frame "57N11" {
                n171 = stacked-sequence {
                  tunnel: w236 -> [w239 w265]
                  tunnel: w235 -> [w238 _]
                  frame #0 {
                    n172 = global read "Meas_global.vi" "Remote control"() -> (w237:bool)
                    n173 = case shown="\"1D\"" w239 {
                      tunnel: w238 -> [w241 w254]
                      tunnel: w237 -> [w240 w253]
                      frame "2D" {
                        n174 = while {
                          tunnel: w240 -> [w242]
                          tunnel: w241 -> [w243]
                          stop <- w244 continue-if-true
                          n175 = stacked-sequence {
                            tunnel: [_ _ w250] -> w244
                            tunnel: w243 -> [w245 w247 _]
                            tunnel: w242 -> [_ _ w249]
                            frame #0 {
                              w246 = "1"  # BSA Number
                              n176 = call "Control_BSA_setup.vi"("setup"=w245, "BSA number"=w246) -> ()  [unwired: 14 out]
                            }
                            frame #1 {
                              w248 = "2"  # BSA Number
                              n177 = call "Control_BSA_setup.vi"("setup"=w247, "BSA number"=w248) -> ()  [unwired: 14 out]
                            }
                            frame #2 {
                              n178 = case shown="False" w249 {
                                tunnel: [w251 FALSE ("ok")] -> w250
                                frame False {
                                n179 = call "BSA_setup_check.vi"() -> ("ok"=w251:bool)
                                }
                                frame True {
                                }
                              }
                            }
                          }
                        }
                      }
                      frame "1D" {
                        n180 = stacked-sequence {
                          tunnel: w254 -> [w255 _]
                          tunnel: w253 -> [_ _]
                          frame #0 {
                            w256 = "1"  # BSA Number
                            n181 = call "Control_BSA_setup.vi"("setup"=w255, "BSA number"=w256) -> ()  [unwired: 14 out]
                          }
                          frame #1 {
                            n182 = global read "LDA_meas_global_2.vi" "BSA2 info"() -> (w257:T27)
                            n183 = Unbundle By Name(w257) -> ("GPIB Address"=w258:string)
                            n184 = call "Set_BSA_Coincidence.vi"("GPIB address"=w258, "Set Coincidence"=enum16{"Slave", "Master", "Private"}."Slave") -> ()  [unwired: 1 in, 5 out]
                          }
                        }
                      }
                    }
                  }
                  frame #1 {
                    n185 = global read "Meas_global.vi" "Remote control"() -> (w263:bool)
                    n186 = Equal?(x=w265, y=enum16{"1D", "2D"}."2D" ("dimensions")) -> (x = y?=w261:bool)
                    n187 = Not(x=w263) -> (.not. x?=w262:bool)
                    n188 = And(x=w262, y=w261) -> (x .and. y?=w260:bool)
                    n189 = case shown="True" w260 {
                      frame False {
                      }
                      frame True {
                        n190 = global read "LDA_meas_global_1.vi" "BSA1 info"() -> (w267:T27)
                        n191 = global read "LDA_meas_global_2.vi" "BSA2 info"() -> (w268:T27)
                        n192 = Build Array(w267, w268) -> (w266:T27[])
                        n193 = for {
                          tunnel: w266 -> [w270] mode=indexing
                          n194 = Unbundle By Name(w270) -> ("GPIB Address"=w269:string)
                          n195 = call "Set_BSA_Coincidence.vi"("GPIB address"=w269, "Set Coincidence"=enum16{"Slave", "Master", "Private"}."Master") -> ()  [unwired: 1 in, 5 out]
                        }
                      }
                    }
                  }
                }
              }
              frame "BSA F60" {
                n196 = disable-structure shown="TARGET_TYPE==Windows" {
                  disable-tunnel: w272 -> [_ w273]
                  frame condition #0 {
                  }
                  frame condition #1 (active) {
                    n197 = while {
                      tunnel: w273 -> [w276]
                      stop <- w274 continue-if-true
                      n198 = call "Edit_BSA_IP.vi"("Show Panel"=w276) -> ("Run LDA Diagnostic Out"=w275:bool)  [unwired: 2 out]
                      n199 = case shown="True" w275 {
                        tunnel: [FALSE w278] -> w274
                        frame False {
                        }
                        frame True {
                          n200 = call "F60_Diagnostic.vi"() -> ("Edit BSA Setup Out"=w278:bool)  [unwired: 11 in]
                        }
                      }
                    }
                  }
                }
              }
            }
          }
        }
      }
      frame #9 {
        w288 = Save_Data."Save No Data" ("File")
        w304 = Post_Process."Take New Data"  # Post Process
        n201 = global read "Trav_pos_global.vi" "Meas Setup Number"() -> (w284:i32)
        n202 = Not Equal?(x=Setup."Run Program" ("setup"), y=w303) -> (x != y?=w289:bool)
        n203 = call "Current_Filepath.vi"("Short_Name"="Res" ("Data Type"), "Filename in"="Results file", "Data Type"="Results") -> ("Filename Out"=w282:path)  [unwired: 1 in, 1 out]
        n204 = global read "Meas_global.vi" "Remote control"() -> (w300:bool)
        n205 = global read "Meas_global.vi" "Post Process"() -> (w291:T2)
        n206 = Equal?(x="File", y=w288) -> (x = y?=w298:bool)
        n207 = case shown="1, Default" w284 {
          tunnel: [w307 w309] -> w285
          tunnel: w282 -> [w307 w316]
          tunnel: w284 -> [_ w317]
          frame 0 {
          }
          frame 1, Default {
            n208 = Add(x=96, y=w317) -> (x+y=w319:i32)
            n209 = Build Array(w319) -> (w320:i32[])
            n210 = Strip Path(path=w316) -> (stripped path=w310:path, name=w315:string)
            n211 = Byte Array To String(unsigned byte array=w320) -> (string=w313:string)
            n212 = call "Add_filename_suffix.vi"("Filename"=w315) -> ("Original Suffix"=w312:string, "Base name"=w314:string)  [unwired: 1 in, 2 out]
            n213 = Format Into String(format string="%s_%s%s", w314, w313, w312) -> (resulting string=w311:string)  [unwired: 2 in, 1 out]
            n214 = Build Path(base path=w310, name or relative path=w311) -> (appended path=w309:path)
          }
        }
        n215 = Equal?(x=w291, y=w304) -> (x = y?=w290:bool)
        n216 = And(x=w300, y=w290) -> (x .and. y?=w296:bool)
        n217 = Compound Arithmetic op=AND(w298, invert w300, w290, invert w289) -> (w299:bool)
        n218 = while {
          shift-left: _ -> [w325]
          shift-right: [w322] -> _
          tunnel: "File" -> [w323]
          tunnel: [w326] -> w297
          tunnel: w299 -> [w322]
          stop <- FALSE continue-if-true
          n219 = Compound Arithmetic op=AND(w322, invert w325) -> (w324:bool)
          n220 = case shown="False" w324 {
            tunnel: [w327 w330] -> w326
            tunnel: w323 -> [w327 _]
            frame False {
            }
            frame True {
              n221 = Two Button Dialog(message="Do you wish to save the data?", 1:"Save Data" ("F button name (\"Cancel\")"), 2:"Save No Data" ("T button name (\"OK\")")) -> (T button?=w331:bool)
              n222 = Select(t=Save_Data."Save No Data" ("File"), s=w331, f=Save_Data."Save Data" ("File")) -> (s? t:f=w330:T5)
            }
          }
        }
        n223 = Equal?(x=w288, y=w297) -> (x = y?=w287:bool)
        n224 = Or(x=w287, y=w289) -> (x .or. y?=w302:bool)
        n225 = case shown="False" w302 {
          tunnel: w285 -> [w346 w354]
          tunnel: [w345 w354] -> w305
          tunnel: "Raw data file" -> [w344 w355]
          tunnel: [w339 w355] -> w294
          tunnel: w303 -> [w343 _]
          tunnel: w297 -> [w342 _]
          tunnel: [w340 T13."Save no data" ("File output")] -> w292
          tunnel: [w341 w352] -> w286
          tunnel: w296 -> [_ w349]
          tunnel: w289 -> [_ w348]
          tunnel: w283 -> [w338 _]
          frame False {
            n226 = call "File_setup.vi"("Measurement is top level?"=w338, "Results file"=w346, "Raw data file"=w344, "setup"=w343, "File"=w342) -> ("Results file output"=w345:path, "Raw data file output"=w339:path, "Raw data option"=w341:enum16{"Save raw data", "Raw data not saved"}, "File output"=w340:T13)
          }
          frame True {
            w350 = enum16{"Save raw data", "Raw data not saved"}."Raw data not saved"  # Raw data option
            n227 = global read "Meas_global.vi" "Raw data option"() -> (w351:enum16{"Save raw data", "Raw data not saved"})
            n228 = Compound Arithmetic op=AND(w349, invert w348) -> (w347:bool)
            n229 = Select(t=w351, s=w347, f=w350) -> (s? t:f=w352:enum16{"Save raw data", "Raw data not saved"})
          }
        }
        n230 = case shown="\"Save raw data\"" w286 {
          tunnel: w294 -> [w335 w337]
          tunnel: [w335 w336] -> w293
          frame "Raw data not saved" {
          }
          frame "Save raw data" {
            n231 = call "Find_Unique_Filename.vi"("Path In"=w337) -> ("Unique Path Out"=w336:path)  [unwired: 1 in, 1 out]
          }
        }
        n232 = local write "Results file"(w305) -> ()
        n233 = global write "Meas_global.vi" "Results file"(w305) -> ()
        n234 = global write "Meas_global.vi" "Raw data option"(w286) -> ()
        n235 = global write "Meas_global.vi" "File"(w292) -> ()
        n236 = global write "Meas_global.vi" "Raw data file"(w293) -> ()
        n237 = local write "Raw data file"(w293) -> ()
        n238 = local write "File"(w297) -> ()
      }
      frame #10 {
        n239 = global read "Meas_global.vi" "Ch & spans"() -> (w358:T28[])
        n240 = local read "Block average display control"() -> (w361:cluster{"Name":string, "Include":bool}[])
        n241 = global read "Meas_global.vi" "LDA data"() -> (w356:enum16{"No LDA data", "Take LDA data"})
        n242 = global read "Meas_global.vi" "Analysis Info cluster"() -> (w357:T22[])
        n243 = global write "Meas_global.vi" "Ch & spans + mod limits"(w358) -> ()
        n244 = case shown="\"No LDA data\"" w356 {
          frame "No LDA data" {
          }
          frame "Take LDA data" {
            n245 = global write "Meas_global.vi" "Time Continuous Across Blocks"(FALSE ("Time Continuous Across Blocks")) -> ()
          }
        }
        n246 = for {
          tunnel: w357 -> [w370] mode=indexing
          tunnel: w361 -> [w369]
          tunnel: [w365] -> w360 mode=indexing
          tunnel: [w366] -> w359 mode=indexing
          i -> [w368]
          n247 = Unbundle By Name(w370) -> ("Symbol"=w365:string)
          n248 = Index Array(array=w369, index=w368) -> (element=w367:cluster{"Name":string, "Include":bool})
          n249 = Bundle By Name(cluster=w367, "Name"=w365) -> (w366:cluster{"Name":string, "Include":bool})
        }
        n250 = local write "Block average display control"(w359) -> ()
        n251 = Build Array (concatenate)("Nothing", w360) -> (w362:string[])
        n252 = property on="Plot 1" class="Ring (strict)"("Strings []"=w362) -> ()  [unwired: 2 in, 2 out]
        n253 = property on="Plot 1" class="Ring (strict)"("Strings []"=w362) -> ()  [unwired: 2 in, 2 out]
        n254 = property on="Plot 2" class="Ring (strict)"("Strings []"=w362) -> ()  [unwired: 2 in, 2 out]
        n255 = property on="Plot 2" class="Ring (strict)"("Strings []"=w362) -> ()  [unwired: 2 in, 2 out]
      }
      frame #11 {
        n256 = global read "Meas_global.vi" "Analysis Info cluster"() -> (w371:T22[])
        n257 = stacked-sequence {
          seq-local: [_ w399 _ _ _] -> [_ _ w430 w485 _]
          seq-local: [_ _ w431 _ _] -> [_ _ _ w484 _]
          seq-local: [_ w398 _ _ _] -> [_ _ w429 _ _]
          seq-local: [w377 _ _ _ _] -> [_ _ w427 _ _]
          seq-local: [w375 _ _ _ _] -> [_ _ w428 _ _]
          seq-local: [w373 _ _ _ _] -> [_ _ w426 _ _]
          tunnel: w371 -> [w380 w402 w432 _ w515]
          frame #0 {
            n258 = for {
              tunnel: w380 -> [w395] mode=indexing
              tunnel: [w394] -> w384
              stop <- w394 stop-if-true
              n259 = Unbundle By Name(w395) -> ("Inst type"=w396:T14)
              n260 = Equal?(x=w396, y=Inst_type."LDA Vel" ("Inst type")) -> (x = y?=w394:bool)
            }
            n261 = global read "Meas_global.vi" "Pre Setup String"() -> (w379:string)
            n262 = global read "Meas_global.vi" "Post Process"() -> (w381:T2)
            n263 = call "Correlation_Setup.vi"("Input string"=w379) -> ("Correlate"=w377:i32[][], "Error?"=w378:bool)
            n264 = Equal?(x=w381, y=Post_Process."Post Process Raw Data File" ("Post Process")) -> (x = y?=w383:bool)
            n265 = Compound Arithmetic op=AND(w384, w383, w378) -> (w375:bool)
            n266 = case shown="\"Correlate without activating panel\"" "Correlate?" {
              tunnel: w377 -> [w389 _ _]
              tunnel: [w387 FALSE FALSE] -> w376
              frame "Cross correlation off" {
                n267 = Array Size(array=w389) -> (size(s)=w391:i32[])
                n268 = Index Array(array=w391, index=0) -> (element=w388:i32)
                n269 = Greater Than 0?(x=w388) -> (x > 0?=w387:bool)
              }
              frame "Show correlation panel" {
              }
              frame "Correlate without activating panel" {
              }
            }
            n270 = Or(x=w376, y=w375) -> (x .or. y?=w374:bool)
            n271 = case shown="False" w374 {
              tunnel: [w385 w386] -> w373
              tunnel: "Correlate?" -> [w385 _]
              frame False {
              }
              frame True {
                w386 = T9."Correlate without activating panel" ("Correlate?")
                n272 = local write "Correlate?"(w386) -> ()
              }
            }
          }
          frame #1 {
            w400 = "RV (WT"
            n273 = String Length(string=w400) -> (length=w401:i32)
            n274 = for {
              tunnel: w402 -> [w421] mode=indexing
              shift-right: [w411] -> w403
              shift-left: i32[] [] -> [w412]
              tunnel: w401 -> [w409]
              tunnel: w400 -> [w407]
              tunnel: [w405] -> w398 mode=indexing
              i -> [w413]
              n275 = Unbundle By Name(w421) -> ("Inst name"=w405:string, "Symbol"=w420:string, "Code name"=w418:string)
              n276 = String Subset(string=w405, length (rest)=w409) -> (substring=w408:string)  [unwired: 1 in]
              n277 = Match Pattern(string=w418, regular expression="Derived") -> (offset past match=w417:i32)  [unwired: 1 in, 3 out]
              n278 = Not Equal?(x=w407, y=w408) -> (x != y?=w406:bool)
              n279 = Less Than 0?(x=w417) -> (x < 0?=w416:bool)
              n280 = Not Equal?(x="Sync", y=w420) -> (x != y?=w415:bool)
              n281 = Compound Arithmetic op=AND(w406, w415, w416) -> (w414:bool)
              n282 = case shown="True" w414 {
                tunnel: w413 -> [_ w425]
                tunnel: w412 -> [w422 w424]
                tunnel: [w422 w423] -> w411
                frame False {
                }
                frame True {
                  n283 = Build Array (concatenate)(w424, w425) -> (w423:i32[])
                }
              }
            }
            n284 = call "Chs_to_Correlate.vi"("Valid Ch to correlate"=w403) -> ("Correlation Pairs"=w399:i32[][])
          }
          frame #2 {
            n285 = case shown="False" w428 {
              tunnel: w432 -> [_ _]
              tunnel: [w435 w480] -> w431
              tunnel: w430 -> [w436 w480]
              tunnel: w429 -> [w440 _]
              tunnel: w427 -> [w434 _]
              tunnel: w426 -> [w433 _]
              frame False {
                n286 = for {
                  tunnel: w436 -> [w465] mode=indexing
                  tunnel: w440 -> [w470]
                  tunnel: [w461] -> w439 mode=indexing
                  tunnel: w434 -> [w466]
                  shift-right: [w462] -> w437
                  shift-left: string[] [] -> [w463]
                  n287 = Index Array(array=w465) -> (element #1=w472:i32, element #2=w471:i32)  [unwired: 2 in]
                  n288 = for {
                    tunnel: w465 -> [w479]
                    tunnel: w466 -> [w478] mode=indexing
                    tunnel: [w477] -> w464
                    stop <- w477 stop-if-true
                    n289 = Equal?(x=w479, y=w478) -> (x = y?=w477:bool)
                  }
                  n290 = Index Array(array=w470, index=w472) -> (element=w469:string)
                  n291 = Index Array(array=w470, index=w471) -> (element=w468:string)
                  n292 = Format Into String(format string="%s & %s", w469, w468) -> (resulting string=w461:string)  [unwired: 2 in, 1 out]
                  n293 = case shown="True" w464 {
                    tunnel: w463 -> [w473 w476]
                    tunnel: [w473 w475] -> w462
                    tunnel: w461 -> [_ w474]
                    frame False {
                    }
                    frame True {
                      n294 = Build Array (concatenate)(w476, w474) -> (w475:string[])
                    }
                  }
                }
                n295 = case shown="\"Show correlation panel\"" w433 {
                  tunnel: w439 -> [_ w448 w452]
                  tunnel: w437 -> [_ w446 w453]
                  tunnel: w436 -> [_ w444 w454]
                  tunnel: [i32[][] [] ("Correlation Pairs") w442 w455] -> w435
                  frame "Cross correlation off" {
                  }
                  frame "Show correlation panel" {
                    n296 = call "Select_Strings.vi"("Available Ch names"=w448, "Message"="Please select Channels to Correlate", "Selector mode"=T15."Zero or more", "Desired Ch names (in)"=w446) -> ("Ch Indicies Choosen"=w443:i32[])  [unwired: 2 in, 2 out]
                    n297 = for {
                      tunnel: w444 -> [w451]
                      tunnel: w443 -> [w450] mode=indexing
                      tunnel: [w449] -> w442 mode=indexing
                      n298 = Index Array(array=w451, index (row)=w450) -> (element=w449:i32[])  [unwired: 1 in]
                    }
                  }
                  frame "Correlate without activating panel" {
                    n299 = for {
                      tunnel: [w460] -> w455 mode=indexing
                      tunnel: w454 -> [w459]
                      tunnel: w453 -> [w458] mode=indexing
                      tunnel: w452 -> [w457]
                      n300 = Search 1D Array(1D array=w457, element=w458) -> (index of element=w456:i32)  [unwired: 1 in]
                      n301 = Index Array(array=w459, index (row)=w456) -> (element=w460:i32[])  [unwired: 1 in]
                    }
                  }
                }
              }
              frame True {
              }
            }
          }
          frame #3 {
            n302 = for {
              shift-right: [w492] -> w482
              shift-left: i32[][] [] -> [w493]
              tunnel: w485 -> [w494]
              tunnel: w484 -> [w491] mode=indexing
              n303 = for {
                tunnel: w494 -> [w509] mode=indexing
                tunnel: w491 -> [w508]
                tunnel: [w507] -> w490
                stop <- w507 stop-if-true
                n304 = Equal?(x=w508, y=w509) -> (x = y?=w507:bool)
              }
              n305 = case shown="True" w490 {
                tunnel: w493 -> [w495 w497]
                tunnel: w491 -> [_ w498]
                tunnel: [w495 w499] -> w492
                frame False {
                }
                frame True {
                  n306 = for {
                    tunnel: w498 -> [w502]
                    tunnel: w497 -> [w501] mode=indexing
                    tunnel: [w500] -> w496
                    stop <- w500 stop-if-true
                    n307 = Equal?(x=w502, y=w501) -> (x = y?=w500:bool)
                  }
                  n308 = case shown="False" w496 {
                    tunnel: w497 -> [w505 w506]
                    tunnel: w498 -> [w504 _]
                    tunnel: [w503 w506] -> w499
                    frame False {
                      n309 = Build Array (concatenate)(w505, w504) -> (w503:i32[][])
                    }
                    frame True {
                    }
                  }
                }
              }
            }
            n310 = global write "Meas_global.vi" "correlate"(w482) -> ()
            n311 = Array Size(array=w482) -> (size(s)=w489:i32[])
            n312 = Index Array(array=w489, index=0) -> (element=w486:i32)
            n313 = Equal To 0?(x=w486) -> (x = 0?=w487:bool)
            n314 = case shown="False" w487 {
              tunnel: [T9."Correlate without activating panel" ("Correlate?") T9."Cross correlation off" ("Correlate?")] -> w481
              frame False {
              }
              frame True {
              }
            }
            n315 = local write "Correlate?"(w481) -> ()
          }
          frame #4 {
            n316 = Array Size(array=w515) -> (size(s)=w513:i32)
            n317 = Initialize Array(T16 {"Weighting"=[], "Time (ms)"=[], "Voltage"=[], "Eng Values"=[]} ("Time Trace"), w513) -> (w512:T29)
            n318 = global write "Meas_global.vi" "Time Trace"(w512) -> ()
          }
        }
      }
      frame #12 {
        n319 = stacked-sequence {
          seq-local: [w522 _] -> [_ w544]
          tunnel: w516 -> [w521 _]
          frame #0 {
            n320 = call "LDA+_An_Analysis_mode.vi"("Second Graph"="Second Graph", "First Graph"="First Graph") -> ("Second Graph out"=w517:T8, "First Graph out"=w519:T8)  [unwired: 6 out]
            n321 = case shown="False" w521 {
              tunnel: [w532 w543] -> w520
              tunnel: w519 -> [w531 w543]
              tunnel: [w530 w542] -> w518
              tunnel: w517 -> [w529 w542]
              frame False {
                w527 = Graph_Type."Show no graph" ("Plot Type")
                n322 = Unbundle By Name(w531) -> ("Save graph"=w533:u16)
                n323 = Unbundle By Name(w529) -> ("Save graph"=w528:u16)
                n324 = case shown="0, Default" w533 {
                  tunnel: [w539 w541] -> w532
                  tunnel: w531 -> [w540 w541]
                  tunnel: w527 -> [w538 _]
                  frame 0, Default {
                    n325 = Bundle By Name(cluster=w540, "Plot Type"=w538) -> (w539:T8)
                  }
                  frame 1 {
                  }
                }
                n326 = case shown="0, Default" w528 {
                  tunnel: [w535 w537] -> w530
                  tunnel: w529 -> [w536 w537]
                  tunnel: w527 -> [w534 _]
                  frame 0, Default {
                    n327 = Bundle By Name(cluster=w536, "Plot Type"=w534) -> (w535:T8)
                  }
                  frame 1 {
                  }
                }
              }
              frame True {
              }
            }
            n328 = local write "Second Graph"(w518) -> ()
            n329 = local write "First Graph"(w520) -> ()
            n330 = global write "Meas_global.vi" "Second Graph"(w518) -> ()
            n331 = global write "Meas_global.vi" "First Graph"(w520) -> ()
            n332 = Unbundle By Name(w518) -> ("Plot Type"=w526:T7)
            n333 = Unbundle By Name(w520) -> ("Plot Type"=w525:T7)
            n334 = Build Array(w525, w526) -> (w522:T7[])
          }
          frame #1 {
            n335 = global read "Meas_global.vi" "Insts for plotting"() -> (w545:u16[][])
            n336 = while {
              tunnel: w545 -> [w552]
              tunnel: w544 -> [w551]
              shift-right: [w549] -> _
              shift-left: _ -> [w547]
              shift-right: [w548] -> _
              shift-left: _ -> [w546]
              stop <- TRUE stop-if-true
              n337 = for {
                tunnel: w552 -> [w558] mode=indexing
                tunnel: w551 -> [w557] mode=indexing
                tunnel: [w556] -> w549 mode=indexing
                tunnel: [w555] -> w548 mode=indexing
                tunnel: w547 -> [w554]
                tunnel: w546 -> [w553]
                i -> [w559]
                n338 = stacked-sequence {
                  seq-local: [w572 _] -> [_ w580]
                  seq-local: [w573 _] -> [_ w579]
                  seq-local: [w560 _] -> [_ w577]
                  tunnel: w559 -> [w569 w581]
                  tunnel: w558 -> [w564 _]
                  tunnel: w557 -> [w566 w578]
                  tunnel: [w564 _] -> w556
                  tunnel: [w566 _] -> w555
                  tunnel: w554 -> [w570 _]
                  tunnel: w553 -> [w568 _]
                  frame #0 {
                    n339 = property on="Plot 1" class="Ring (strict)"() -> ("Strings []"=w571:string[])  [unwired: 2 in, 2 out]
                    n340 = Array To Cluster(array=w564) -> (cluster=w576:T30)
                    n341 = Index Array(array=w570, index (row)=w569) -> (element=w565:u16[])  [unwired: 1 in]
                    n342 = Index Array(array=w568, index=w569) -> (element=w567:T7)
                    n343 = Unbundle(w576) -> ("Insts for plotting[0]"=w575:u16, "Insts for plotting[1]"=w574:u16)
                    n344 = Not Equal?(x=w567, y=w566) -> (x != y?=w563:bool)
                    n345 = Not Equal?(x=w564, y=w565) -> (x != y?=w562:bool[])
                    n346 = Index Array(array=w571, index=w575) -> (element=w572:string)
                    n347 = Index Array(array=w571, index=w574) -> (element=w573:string)
                    n348 = Or Array Elements(Boolean array=w562) -> (logical OR=w561:bool)
                    n349 = Or(x=w561, y=w563) -> (x .or. y?=w560:bool)
                  }
                  frame #1 {
                    n350 = case shown="True" w577 {
                      tunnel: w581 -> [_ w592]
                      tunnel: w580 -> [_ w589]
                      tunnel: w579 -> [_ w588]
                      tunnel: w578 -> [_ w584]
                      frame False {
                      }
                      frame True {
                        n351 = case shown="\"Velocity trace\"" w584 {
                          tunnel: [u8 0 u8 0 u8 0 u8 0 u8 0 u8 1 u8 0] -> w596
                          tunnel: [u8 0 u8 0 u8 0 u8 0 u8 1 u8 1 u8 0] -> w595
                          tunnel: [u8 0 u8 0 u8 0 u8 0 u8 1 u8 1 u8 0] -> w594
                          tunnel: [u8 0 u8 0 u8 0 u8 0 u8 1 u8 0 u8 0] -> w593
                          tunnel: [FALSE TRUE TRUE TRUE TRUE TRUE TRUE] -> w587
                          tunnel: [u8 0 u8 1 u8 1 u8 2 u8 0 u8 0 u8 2] -> w586
                          tunnel: [u8 0 u8 4 u8 1 u8 2 u8 0 u8 0 u8 1] -> w585
                          tunnel: ["" "Time (s)" "Time (s)" "" "" "" ""] -> w583
                          tunnel: ["" "Voltage" "Velocity" "" "" "" ""] -> w582
                          frame "Show no graph" {
                          }
                          frame "Voltage trace" {
                          }
                          frame "Velocity trace" {
                          }
                          frame "Vel histogram" {
                          }
                          frame "Spectrum" {
                          }
                          frame "f.E(f) v Log f" {
                          }
                          frame "Auto-Corr" {
                          }
                        }
                        n352 = case shown="1" w592 {
                          tunnel: w587 -> [w609 w622]
                          tunnel: w596 -> [w608 w621]
                          tunnel: w595 -> [w607 w620]
                          tunnel: w594 -> [w606 w619]
                          tunnel: w593 -> [w605 w618]
                          tunnel: u32 0 -> [w604 w617]
                          tunnel: u32 1 -> [w603 w615]
                          tunnel: w589 -> [w602 w616]
                          tunnel: w588 -> [w601 w614]
                          tunnel: w586 -> [w600 w613]
                          tunnel: w585 -> [w599 w612]
                          tunnel: w583 -> [w598 w611]
                          tunnel: w582 -> [w597 w610]
                          frame 0, Default {
                            n353 = property on="First plot" class="XYGraph (strict)"("Visible"=w609, "X Scale.Format & Precision:Format"=w608, "X Scale.Mapping Mode"=w607, "Y Scale.Format & Precision:Format"=w606, "Y Scale.Mapping Mode"=w605, "Active Plot"=w604, "Plot.Plot Name"=w602, "Active Plot"=w603, "Plot.Plot Name"=w601, "X Scale.Format & Precision:Precision"=w600, "Y Scale.Format & Precision:Precision"=w599, "XScale.NameLbl.Text"=w598, "YScale.NameLbl.Text"=w597) -> ()  [unwired: 2 in, 2 out]
                          }
                          frame 1 {
                            n354 = property on="2nd plot" class="XYGraph (strict)"("Visible"=w622, "X Scale.Format & Precision:Format"=w621, "X Scale.Mapping Mode"=w620, "Y Scale.Format & Precision:Format"=w619, "Y Scale.Mapping Mode"=w618, "Active Plot"=w617, "Plot.Plot Name"=w616, "Active Plot"=w615, "Plot.Plot Name"=w614, "X Scale.Format & Precision:Precision"=w613, "Y Scale.Format & Precision:Precision"=w612, "XScale.NameLbl.Text"=w611, "YScale.NameLbl.Text"=w610) -> ()  [unwired: 2 in, 2 out]
                          }
                        }
                      }
                    }
                  }
                }
              }
            }
          }
        }
      }
      frame #13 {
        n355 = local read "Second Graph"() -> (w697:T8)
        n356 = local read "First Graph"() -> (w696:T8)
        n357 = Unbundle By Name(w696) -> ("Plot 1"=w689:u16, "Plot 2"=w690:u16)
        n358 = Unbundle By Name(w697) -> ("Plot 1"=w691:u16, "Plot 2"=w692:u16)
        n359 = Build Array(w689, w690) -> (w693:u16[])
        n360 = Build Array(w691, w692) -> (w694:u16[])
        n361 = global read "Meas_global.vi" "Analysis Info cluster"() -> (w698:T22[])
        n362 = Decrement(x=w693) -> (x-1=w687:u16[])
        n363 = Decrement(x=w694) -> (x-1=w695:u16[])
        n364 = for {
          tunnel: w698 -> [w706]
          tunnel: w687 -> [w705] mode=indexing
          shift-right: [w699] -> _
          shift-left: u32 0 -> [w701]
          i -> [w700]
          n365 = Index Array(array=w706, index=w705) -> (element=w707:T22)
          n366 = Unbundle By Name(w707) -> ("Colour"=w702:u32)
          n367 = Equal?(x=w702, y=w701) -> (x = y?=w704:bool)
          n368 = Select(t=u32 13434624, s=w704, f=w702) -> (s? t:f=w699:u32)
          n369 = property on="First plot" class="XYGraph (strict)"("Active Plot"=w700, "Plot.Plot Color"=w699, "Plot.Fill/Point Color"=w699) -> ()  [unwired: 2 in, 2 out]
        }
        n370 = for {
          tunnel: w698 -> [w715]
          tunnel: w695 -> [w714] mode=indexing
          shift-right: [w710] -> _
          shift-left: u32 0 -> [w708]
          i -> [w713]
          n371 = Index Array(array=w715, index=w714) -> (element=w716:T22)
          n372 = Unbundle By Name(w716) -> ("Colour"=w709:u32)
          n373 = Equal?(x=w709, y=w708) -> (x = y?=w712:bool)
          n374 = Select(t=u32 13434624, s=w712, f=w709) -> (s? t:f=w710:u32)
          n375 = property on="2nd plot" class="XYGraph (strict)"("Active Plot"=w713, "Plot.Plot Color"=w710, "Plot.Fill/Point Color"=w710) -> ()  [unwired: 2 in, 2 out]
        }
      }
      frame #14 {
        n376 = global read "DataTranslation_global.vi" "Different Sampling Freq per block"() -> (w720:bool)
        n377 = global read "Meas_global.vi" "Remote control"() -> (w727:bool)
        n378 = global read "Meas_global.vi" "Post Process"() -> (w730:T2)
        n379 = global read "Meas_global.vi" "PWA Data"() -> (w721:T31)
        n380 = case shown="\"One Ch PWA\"" w721 {
          tunnel: [w731 w736] -> w723
          frame "No PWA Data" {
            n381 = local read "Desired Sampling freq (Hz)"() -> (w733:dbl)
            n382 = local read "No of samples"() -> (w732:i32)
            n383 = Divide(x=w732, y=w733) -> (x/y=w731:dbl)
          }
          frame "One Ch PWA" {
            n384 = local read "No of samples"() -> (w734:i32)
            n385 = global read "PWAtasksGLOBAL.vi" "PWA Freq. (Hz)"() -> (w735:dbl)
            n386 = global write "PWAtasksGLOBAL.vi" "PWA No. of Samples"(w734) -> ()
            n387 = Divide(x=w734, y=w735) -> (x/y=w736:dbl)
          }
        }
        n388 = Equal?(x=Setup."Run Program" ("setup"), y=w725) -> (x = y?=w718:bool)
        n389 = global read "Meas_global.vi" "Averaging time (min)"() -> (w726:dbl)
        n390 = Equal?(x=Post_Process."Take New Data" ("Post Process"), y=w730) -> (x = y?=w719:bool)
        n391 = And(x=w719, y=w718) -> (x .and. y?=w717:bool)
        n392 = Compound Arithmetic op=AND(invert w720, invert w722, invert w727, w717) -> (w728:bool)
        n393 = case shown="True" w728 {
          tunnel: w726 -> [_ w743]
          tunnel: w723 -> [_ w742]
          frame False {
          }
          frame True {
            n394 = Multiply(x=w743, y=60.0) -> (x*y=w739:dbl)
            n395 = Divide(x=w739, y=w742) -> (x/y=w738:dbl)
            n396 = Round Toward +Infinity(x=w738) -> (ceil(x): smallest int >= x=w737:dbl)
            n397 = To Long Integer(number=w737) -> (32bit integer=w741:i32)
            n398 = global write "Meas_global.vi" "Requested No of blocks"(w741) -> ()
            n399 = local write "No of Blocks"(w741) -> ()
          }
        }
      }
      frame #15 {
        n400 = case shown="\"Run Program\"" w744 {
          frame "Run Program" {
            n401 = call "Read_calibration_files.vi"() -> ()  [unwired: 1 out]
            n402 = global write "Meas_global.vi" "Repeat Measurement?"(FALSE ("Repeat Measurement?")) -> ()
          }
          frame "Show Setup", Default {
          }
        }
      }
      frame #16 {
        n403 = global read "Meas_global.vi" "Raw data option"() -> (w750:enum16{"Save raw data", "Raw data not saved"})
        n404 = Get Date/Time In Seconds() -> (seconds since 1Jan1904=w746:timestamp)
        n405 = To Double Precision Float(number=w746) -> (double precision float=w748:dbl)
        n406 = global read "Meas_global.vi" "Post Process"() -> (w749:T2)
        n407 = case shown="\"Setup Front Panel\"" w751 {
          tunnel: w750 -> [w753 _ _ _]
          tunnel: w749 -> [w752 _ w794 w803]
          frame "Run Program" {
            n408 = case shown="\"Take New Data\"" w752 {
              tunnel: w753 -> [w763 _]
              frame "Take New Data" {
                n409 = case shown="\"Raw data not saved\"" w763 {
                  frame "Save raw data" {
                  }
                  frame "Raw data not saved" {
                    w771 = FALSE  # Lock File
                    w768 = FALSE  # advisory dialog? (display:T)
                    w767 = FALSE  # append to file? (new file:F)
                    n410 = global read "Meas_global.vi" "Remote control"() -> (w769:bool)
                    n411 = call "Create_setup_string.vi"() -> ("Setup String"=w772:string)  [unwired: 1 out]
                    n412 = case shown="False" w769 {
                      tunnel: ["Current_Setup.xls" ("Setup filename") w774] -> w764
                      frame False {
                      }
                      frame True {
                        n413 = local read "Setup filename"() -> (w774:string)
                      }
                    }
                    n414 = call "Add_length_to_string.vi"("String in"=w772) -> ("String out"=w770:string)
                    n415 = call "Setup_Filepath.vi"("Setup File Type"=Setup_Filetype."Measurement Setups", "Filename in"=w764) -> ("Filename Out"=w765:path)  [unwired: 1 out]
                    n416 = call "Write_Characters_To_File.vi"("file path (dialog if empty)"=w765, "advisory dialog? (display:T)"=w768, "character string"=w770, "append to file? (new file:F)"=w767, "Lock File"=w771) -> ()  [unwired: 4 out]
                  }
                }
                n417 = global read "Meas_global.vi" "Requested No of samples"() -> (w757:i32)
                n418 = global read "Meas_global.vi" "Requested Sampling rate"() -> (w760:dbl)
                n419 = global read "Meas_global.vi" "Requested No of blocks"() -> (w756:i32)
                n420 = Divide(x=w757, y=w760) -> (x/y=w759:dbl)
                n421 = Multiply(x=w756, y=w759) -> (x*y=w755:dbl)
                n422 = Add(x=w755, y=120.0) -> (x+y=w754:dbl)
                n423 = call "Program_Active_Client.vi"("Mode"=enum16{"Program Active", "Traverse Level State"}."Program Active", "Time till next contact (Sec)"=w754, "Traverse level State"=Traverse_Level_State."Running") -> ()  [unwired: 3 out]
              }
              frame "Post Process Raw Data File" {
              }
            }
          }
          frame "Save Current Setup" {
            n424 = stacked-sequence {
              seq-local: [w777 _] -> [_ w780]
              seq-local: [w776 _] -> [_ w779]
              frame #0 {
                w778 = FALSE  # Save New File?
                n425 = call "Save_current_setup.vi"("Save New File?"=w778, "Setup File Type"=Setup_Filetype."Measurement Setups") -> ("Cancelled?"=w776:bool, "Saved filepath"=w777:path)  [unwired: 2 out]
              }
              frame #1 {
                n426 = case shown="False" w779 {
                  tunnel: w780 -> [w786 _]
                  frame False {
                    w783 = "Initial Probe positions" ("File Label")
                    w791 = FALSE  # append to file? (new file:F)
                    w792 = FALSE  # advisory dialog? (display:T)
                    w793 = FALSE  # Lock File
                    n427 = call "Input_Instrument_Positions.vi"("Filepath to Save"=w786) -> ("Output string"=w785:string)  [unwired: 1 out]
                    n428 = call "Create_setup_string.vi"() -> ("Setup String"=w784:string)  [unwired: 1 out]
                    n429 = call "Get_string_subset.vi"("String to split"=w785, "File Label"=w783) -> ("Output string"=w782:string)  [unwired: 2 in, 1 out]
                    n430 = call "Replace_data_in_Label_str.vi"("New data string"=w782, "Input string"=w784, "Variable name"=w783) -> ("Appended string"=w781:string)
                    n431 = call "Replace_data_in_setup_string.vi"("New data string"="", "Input string"=w781, "Variable name"="Comments") -> ("Appended string"=w787:string)
                    n432 = call "Add_length_to_string.vi"("String in"=w787) -> ("String out"=w790:string)
                    n433 = call "Write_Characters_To_File.vi"("file path (dialog if empty)"=w786, "advisory dialog? (display:T)"=w792, "character string"=w790, "append to file? (new file:F)"=w791, "Lock File"=w793) -> ()  [unwired: 4 out]
                  }
                  frame True {
                  }
                }
              }
            }
          }
          frame "Show Setup" {
            n434 = case shown="\"Take New Data\"" w794 {
              frame "Take New Data" {
                w799 = FALSE  # append to file? (new file:F)
                w800 = FALSE  # advisory dialog? (display:T)
                w801 = FALSE  # Lock File
                n435 = call "Create_setup_string.vi"() -> ("Setup String"=w802:string)  [unwired: 1 out]
                n436 = call "Add_length_to_string.vi"("String in"=w802) -> ("String out"=w798:string)
                n437 = call "Setup_Filepath.vi"("Setup File Type"=Setup_Filetype."Measurement Setups", "Filename in"="Current_Setup.xls" ("Setup filename")) -> ("Filename Out"=w796:path)  [unwired: 1 out]
                n438 = call "Write_Characters_To_File.vi"("file path (dialog if empty)"=w796, "advisory dialog? (display:T)"=w800, "character string"=w798, "append to file? (new file:F)"=w799, "Lock File"=w801) -> ()  [unwired: 4 out]
              }
              frame "Post Process Raw Data File" {
              }
            }
          }
          frame "Setup Front Panel" {
            n439 = case shown="\"Take New Data\"" w803 {
              frame "Take New Data" {
                w808 = FALSE  # append to file? (new file:F)
                w809 = FALSE  # advisory dialog? (display:T)
                w810 = FALSE  # Lock File
                n440 = call "Create_setup_string.vi"() -> ("Setup String"=w811:string)  [unwired: 1 out]
                n441 = call "Add_length_to_string.vi"("String in"=w811) -> ("String out"=w807:string)
                n442 = call "Setup_Filepath.vi"("Setup File Type"=Setup_Filetype."Measurement Setups", "Filename in"="Current_Setup.xls" ("Setup filename")) -> ("Filename Out"=w805:path)  [unwired: 1 out]
                n443 = call "Write_Characters_To_File.vi"("file path (dialog if empty)"=w805, "advisory dialog? (display:T)"=w809, "character string"=w807, "append to file? (new file:F)"=w808, "Lock File"=w810) -> ()  [unwired: 4 out]
              }
              frame "Post Process Raw Data File" {
              }
            }
          }
        }
        n444 = global write "Meas_global.vi" "Actual Measurement time (min)"(0.0 ("Max Measurement time (min)")) -> ()
      }
      frame #17 {
        n445 = global read "Dynamic_call_global.ph.vi" "Initial Plug Ins"() -> (w813:string[])
        n446 = global read "Dynamic_call_global.ph.vi" "Initial Plug Ins Extra"() -> (w814:string[])
        n447 = Build Array (concatenate)(w814, w813) -> (w812:string[])
        n448 = Array Size(array=w812) -> (size(s)=w816:i32)
        n449 = Greater Than 0?(x=w816) -> (x > 0?=w815:bool)
        n450 = case shown="True" w815 {
          tunnel: w812 -> [_ w817]
          frame False {
          }
          frame True {
            n451 = stacked-sequence {
              tunnel: w817 -> [w819 _]
              frame #0 {
                n452 = global read "Meas_global.vi" "Post Process"() -> (w821:T2)
                n453 = call "Plug_in_Directories.vi"() -> ("Initial"=w818:path)  [unwired: 3 out]
                n454 = Equal?(x=w821, y=Post_Process."Post Process Raw Data File" ("Post Process")) -> (x = y?=w820:bool)
                n455 = for {
                  tunnel: w820 -> [w827]
                  tunnel: w819 -> [w824] mode=indexing
                  tunnel: w818 -> [w823]
                  w834 = FALSE  # Dialog Box (T)
                  n456 = Build Path(base path=w823, name or relative path=w824) -> (appended path=w825:path)
                  n457 = Open VI Reference(vi path=w825) -> (vi reference=w832:refnum<vi>, error out=w831:errorcluster)  [unwired: 2 in, 3 out]
                  n458 = property class="VI"(reference=w832, error in=w831, "Front Panel Window:Open"=TRUE ("Wait until done")) -> (reference out=w830:refnum<vi>, error out=w829:errorcluster)
                  n459 = invoke class="VI" method="Run VI"(reference=w830, error in=w829, "Wait until done"=w827, "Auto Dispose Ref"=FALSE) -> (reference out=w837:refnum<vi>, error out=w836:errorcluster)  [unwired: 1 in, 3 out]
                  n460 = Close Reference(reference=w837, error in (no error)=w836) -> (error out=w835:errorcluster)
                  n461 = call "EnFlo_Error_Handler.vi"("error in (no error)"=w835, "Error Type"="Launching Initial Plug In", "Dialog Box (T)"=w834) -> ()  [unwired: 3 out]
                }
              }
              frame #1 {
                n462 = global read "Meas_global.vi" "Requested No of blocks"() -> (w839:i32)
                n463 = global read "Meas_global.vi" "Comments"() -> (w838:string)
                n464 = local write "Comments"(w838) -> ()
                n465 = local write "No of Blocks"(w839) -> ()
              }
            }
          }
        }
      }
      frame #18 {
        n466 = case shown="\"Run Program\"" w844 {
          tunnel: w841 -> [w847 _]
          tunnel: w843 -> [_ w1000]
          tunnel: w842 -> [w846 _]
          tunnel: w840 -> [w845 _]
          frame "Run Program" {
            n467 = while {
              tunnel: w847 -> [w853]
              tunnel: w846 -> [_]
              tunnel: w845 -> [w852]
              shift-right: [w851] -> _
              shift-left: _ -> [w850]
              shift-right: [w848] -> _
              shift-left: _ -> [w849]
              i -> [w854]
              stop <- w855 stop-if-true
              n468 = Increment(x=w854) -> (x+1=w856:i32)
              n469 = stacked-sequence {
                seq-local: [_ _ _ _ _ "Block average display control" _ _ _ _] -> [_ _ _ _ _ _ w945 _ _ _]
                seq-local: [_ _ _ _ _ _ w943 _ _ _] -> [_ _ _ _ _ _ _ w961 _ _]
                seq-local: [_ _ _ _ w926 _ _ _ _ _] -> [_ _ _ _ _ _ _ _ _ w993]
                seq-local: [_ w886 _ _ _ _ _ _ _ _] -> [_ _ w919 _ _ _ _ _ _ _]
                seq-local: [_ _ w917 _ _ _ _ _ _ _] -> [_ _ _ _ _ _ _ _ _ w996]
                seq-local: [w864 _ _ _ _ _ _ _ _ _] -> [_ w885 _ _ _ _ _ _ _ _]
                seq-local: [w858 _ _ _ _ _ _ _ _ _] -> [_ w880 _ _ _ _ _ _ _ _]
                seq-local: [w857 _ _ _ _ _ _ _ _ _] -> [_ w882 _ _ _ _ _ _ _ _]
                tunnel: w856 -> [w870 _ w918 _ _ w935 _ _ _ w997]
                tunnel: [_ _ w917 _ _ _ _ _ _ _] -> w855
                tunnel: w853 -> [_ _ _ _ w925 _ _ _ _ _]
                tunnel: w852 -> [_ _ _ _ _ _ _ _ _ _]
                tunnel: [_ w884 _ _ _ _ _ _ _ _] -> w851
                tunnel: w850 -> [w863 w883 _ _ _ _ _ _ _ _]
                tunnel: w849 -> [w862 w879 _ _ _ _ _ _ _ _]
                tunnel: [_ w881 _ _ _ _ _ _ _ _] -> w848
                frame #0 {
                  w878 = string[] [] ("Plug in titles")
                  n470 = global read "Trav_pos_global.vi" "Trav Last Moved"() -> (w857:timestamp)
                  n471 = global read "Trav_pos_global.vi" "Top level setup filename"() -> (w858:path)
                  n472 = Not Equal?(x=w863, y=w857) -> (x != y?=w860:bool)
                  n473 = Not Equal?(x=w858, y=w862) -> (x != y?=w861:bool)
                  n474 = Or(x=w861, y=w860) -> (x .or. y?=w859:bool)
                  n475 = global read "Meas_global.vi" "Raw data option"() -> (w872:enum16{"Save raw data", "Raw data not saved"})
                  n476 = global read "Preference_global.vi" "Log Cameras if available"() -> (w873:bool)
                  n477 = global read "Meas_global.vi" "Post Process"() -> (w876:T2)
                  n478 = global read "Trav_pos_global.vi" "Meas Setup Number"() -> (w867:i32)
                  n479 = global write "Meas_global.vi" "Current Block No"(w870) -> ()
                  n480 = Equal?(x=enum16{"Save raw data", "Raw data not saved"}."Save raw data" ("Raw data option"), y=w872) -> (x = y?=w868:bool)
                  n481 = Equal?(x=1, y=w870) -> (x = y?=w869:bool)
                  n482 = Equal?(x=Post_Process."Take New Data" ("Post Process"), y=w876) -> (x = y?=w874:bool)
                  n483 = Less?(x=w867, y=2) -> (x < y?=w865:bool)
                  n484 = Compound Arithmetic op=AND(w859, w873, w874, w868, w869, w865) -> (w864:bool)
                  n485 = global write "Dynamic_call_global.ph.vi" "Plug in values"(w878) -> ()
                  n486 = global write "Dynamic_call_global.ph.vi" "Plug in titles"(w878) -> ()
                  "Current Block No" <- w870
                }
                frame #1 {
                  n487 = case shown="True" w885 {
                    tunnel: [w889 w895] -> w884
                    tunnel: w883 -> [w889 w894]
                    tunnel: w882 -> [_ w893]
                    tunnel: [w888 w892] -> w881
                    tunnel: w880 -> [_ w891]
                    tunnel: w879 -> [w888 w890]
                    frame False {
                    }
                    frame True {
                      n488 = global read "Preference_global.vi" "Rig Setup"() -> (w896:string)
                      n489 = case shown="\"EnFlo_Tunnel\"" w896 {
                        tunnel: [w898 w900] -> w895
                        tunnel: w894 -> [w898 _]
                        tunnel: w893 -> [_ w900]
                        tunnel: [w897 w899] -> w892
                        tunnel: w891 -> [_ w899]
                        tunnel: w890 -> [w897 _]
                        frame "False", Default {
                        }
                        frame "EnFlo_Tunnel" {
                          n490 = Current VI's Path() -> (path=w911:path)
                          n491 = Strip Path(path=w911) -> (stripped path=w910:path)  [unwired: 1 out]
                          n492 = Build Path(base path=w910, name or relative path="Utilities") -> (appended path=w913:path)
                          n493 = Build Path(base path=w913, name or relative path="Image acquisition and processing") -> (appended path=w914:path)
                          n494 = Build Path(base path=w914, name or relative path="Call_Video_Still_with_Averaging.vi") -> (appended path=w909:path)
                          n495 = Open VI Reference(type specifier VI Refnum (for type only)=refnum<vi> refnum, vi path=w909, options=256) -> (vi reference=w905:refnum<vi>, error out=w906:errorcluster)  [unwired: 3 in]
                          n496 = call-by-ref "Start Asynchronous Call"(reference=w905, error in=w906) -> (error out=w902:errorcluster)  [unwired: 1 in, 2 out]
                          n497 = call-by-ref "Wait On Asynchronous Call"(reference=w905, error in=w906) -> (reference out=w904:refnum<vi>, error out=w903:errorcluster)  [unwired: 1 in, 1 out]
                          n498 = Close Reference(reference=w904, error in (no error)=w903) -> (error out=w901:errorcluster)
                          n499 = Merge Errors(w902, w901) -> ()  [unwired: 1 out]
                        }
                      }
                    }
                  }
                  n500 = call "Get_data.vi"() -> ("EOF? and Error status"=w886:bool, "Block Header"=w887:string)  [unwired: 10 out]
                  n501 = global write "Plug_in_data_global.vi" "Block Header"(w887) -> ()
                }
                frame #2 {
                  n502 = global write "Meas_global.vi" "Requested No of blocks"("No of Blocks") -> ()
                  n503 = Less Or Equal?(x="No of Blocks", y=w918) -> (x <= y?=w921:bool)
                  n504 = Compound Arithmetic op=OR(w919, w921) -> (w917:bool)
                  n505 = case shown="True" w917 {
                    tunnel: w918 -> [_ w922]
                    frame False {
                    }
                    frame True {
                      n506 = global write "Meas_global.vi" "Requested No of blocks"(w922) -> ()
                      n507 = local write "No of Blocks"(w922) -> ()
                    }
                  }
                  n508 = global write "Meas_global.vi" "Processing last block?"(w917) -> ()
                  n509 = global write "PWAtasksGLOBAL.vi" "STOP"(w917) -> ()
                }
                frame #3 {
                  n510 = call "Text_without_format.vi"("Input string"="Comments") -> ("Output string"=w923:string)
                  n511 = local write "Comments"(w923) -> ()
                  n512 = global write "Meas_global.vi" "Comments"(w923) -> ()
                }
                frame #4 {
                  n513 = call "Process_data.vi"("Measurement top level?"=w925) -> ("Vel stat display"=→"Statistics":string[][], "First Plot data Cluster"=→"First plot":cluster{"X array":dbl[], "Y array":dbl[]}[], "Second Plot Data Cluster"=→"2nd plot":cluster{"X array":dbl[], "Y array":dbl[]}[], "Max Measurement time up"=w926:bool)  [unwired: 5 in]
                }
                frame #5 {
                  n514 = global read "Meas_global.vi" "Actual Measurement time (min)"() -> (→"Measurement time (min)":dbl)
                  n515 = global read "Meas_global.vi" "Actual Sampling rate (Hz)"() -> (→"Actual Sampling freq":dbl)
                  n516 = call "Display_blocks.vi"("Block No"=w935, "Block average display"="Block average display control") -> ("u^4"=→"u^4":dbl[][], "u^3"=→"u^3":dbl[][], "uv"=→"uv":dbl[][], "u^2"=→"u^2" →"Array u^2":dbl[][], "U"=→"U" →"Array U":dbl[][])  [unwired: 4 out]
                }
                frame #6 {
                  n517 = global read "Meas_global.vi" "Analysis Info cluster"() -> (w944:T22[])
                  n518 = global read "Meas_global.vi" "Diagnostic info"() -> (w942:string[][])
                  n519 = for {
                    tunnel: w945 -> [w960] mode=indexing
                    tunnel: w944 -> [w957] mode=indexing
                    tunnel: [w959] -> w943 mode=indexing if=w958
                    tunnel: [w947] -> w941 mode=indexing
                    tunnel: [w946] -> w940 mode=indexing
                    n520 = Unbundle By Name(w957) -> ("Colour"=w959:u32)
                    n521 = Unbundle By Name(w960) -> ("Include"=w958:bool)
                    n522 = Unbundle By Name(w957) -> ("Inst name"=w951:string, "Av Sampling Rate"=w953:dbl, "Av No of Samples"=w950:dbl)
                    n523 = Format Into String(format string="%s Freq Hz", w951) -> (resulting string=w955:string)  [unwired: 2 in, 1 out]
                    n524 = Format Into String(format string="%s Samples per block", w951) -> (resulting string=w948:string)  [unwired: 2 in, 1 out]
                    n525 = Number To Decimal String(number=w953) -> (decimal integer string=w954:string)  [unwired: 1 in]
                    n526 = Number To Decimal String(number=w950) -> (decimal integer string=w949:string)  [unwired: 1 in]
                    n527 = Build Array(w955, w954) -> (w947:string[])
                    n528 = Build Array(w948, w949) -> (w946:string[])
                  }
                  n529 = Build Array (concatenate)(w942, w941, w940) -> (→"Diagnostic info":string[][])
                }
                frame #7 {
                  n530 = for {
                    tunnel: w961 -> [w962] mode=indexing
                    i -> [w963]
                    n531 = property on="U" class="WFGraph (strict)"("Active Plot"=w963, "Plot.Plot Color"=w962, "Plot.Fill/Point Color"=w962) -> ()  [unwired: 2 in, 2 out]
                    n532 = property on="u^3" class="WFGraph (strict)"("Active Plot"=w963, "Plot.Plot Color"=w962, "Plot.Fill/Point Color"=w962) -> ()  [unwired: 2 in, 2 out]
                    n533 = property on="u^4" class="WFGraph (strict)"("Active Plot"=w963, "Plot.Plot Color"=w962, "Plot.Fill/Point Color"=w962) -> ()  [unwired: 2 in, 2 out]
                    n534 = property on="u^2" class="WFGraph (strict)"("Active Plot"=w963, "Plot.Plot Color"=w962, "Plot.Fill/Point Color"=w962) -> ()  [unwired: 2 in, 2 out]
                  }
                }
                frame #8 {
                  n535 = case shown="True" "Pause" {
                    frame False {
                    }
                    frame True {
                      n536 = global read "Meas_global.vi" "Post Process"() -> (w965:T2)
                      n537 = case shown="\"Post Process Raw Data File\"" w965 {
                        frame "Take New Data" {
                          n538 = call "Program_Active_Client.vi"("Mode"=enum16{"Program Active", "Traverse Level State"}."Program Active", "Time till next contact (Sec)"=12000.0, "Traverse level State"=Traverse_Level_State."Running") -> ()  [unwired: 3 out]
                          n539 = while {
                            i -> [w972]
                            stop <- w973 continue-if-true
                            n540 = Quotient & Remainder(x=w972, y=10) -> (x-y*floor(x/y)=w970:i32)  [unwired: 1 out]
                            n541 = Equal To 0?(x=w970) -> (x = 0?=w969:bool)
                            n542 = stacked-sequence {
                              seq-local: [_ w975 _ _] -> [_ _ w977 _]
                              tunnel: [_ w975 _ _] -> w973
                              tunnel: w969 -> [_ _ _ w979]
                              frame #0 {
                                "Pause message" <- "Measurement Program Paused!!!!" ("Pause message")
                              }
                              frame #1 {
                                n543 = global write "Trav_pos_global.vi" "Paused During Row?"(TRUE ("Paused During Row?")) -> ()
                                n544 = local read "Pause"() -> (w975:bool)
                              }
                              frame #2 {
                                n545 = property on="Pause message" class="Str"("Blinking"=w977, "Visible"=w977) -> ()  [unwired: 2 in, 2 out]
                                n546 = Wait Until Next ms Multiple(millisecond multiple=u32 1000) -> ()  [unwired: 1 out]
                              }
                              frame #3 {
                                n547 = case shown="False" w979 {
                                frame False {
                                }
                                frame True {
                                n548 = Current VI's Path() -> (path=w980:path)
                                n549 = call "Bring_to_front.vi"("path"=w980) -> ()
                                }
                                }
                              }
                            }
                          }
                        }
                        frame "Post Process Raw Data File" {
                          n550 = stacked-sequence {
                            seq-local: [_ w983 _ _] -> [_ _ _ w990]
                            frame #0 {
                              n551 = property on="PP next block" class="Bool (strict)"("Visible"=TRUE) -> ()  [unwired: 2 in, 2 out]
                              n552 = local write "PP next block"(FALSE ("PP next block")) -> ()
                            }
                            frame #1 {
                              n553 = while {
                                tunnel: [w987] -> w983
                                stop <- w984 stop-if-true
                                n554 = local read "stop"() -> (w987:bool)
                                n555 = local read "Pause"() -> (w985:bool)
                                n556 = Compound Arithmetic op=OR(w987, "PP next block", invert w985) -> (w984:bool)
                                n557 = case shown="False" w984 {
                                frame False {
                                n558 = Wait (ms)(milliseconds to wait=u32 200) -> ()  [unwired: 1 out]
                                }
                                frame True {
                                }
                                }
                              }
                            }
                            frame #2 {
                              n559 = property on="PP next block" class="Bool (strict)"("Visible"=FALSE) -> ()  [unwired: 2 in, 2 out]
                            }
                            frame #3 {
                              n560 = Stop(stop? (T)=w990) -> ()
                            }
                          }
                        }
                      }
                    }
                  }
                }
                frame #9 {
                  n561 = global read "Meas_global.vi" "stop"() -> (w991:bool)
                  n562 = Compound Arithmetic op=OR("stop", w993, w991) -> (w992:bool)
                  n563 = Compound Arithmetic op=AND(w992, invert w996) -> (w995:bool)
                  n564 = case shown="True" w995 {
                    tunnel: w997 -> [_ w999]
                    frame False {
                    }
                    frame True {
                      n565 = Increment(x=w999) -> (x+1=w998:i32)
                      n566 = local write "No of Blocks"(w998) -> ()
                      n567 = global write "Meas_global.vi" "Requested No of blocks"(w998) -> ()
                    }
                  }
                }
              }
            }
          }
          frame "Setup Front Panel", Default {
            n568 = stacked-sequence {
              seq-local: [w1001 _ _ _ _ _ _] -> [_ _ _ _ _ w1075 _]
              seq-local: [_ w1007 _ _ _ _ _] -> [_ _ _ _ _ w1074 _]
              seq-local: [_ _ _ w1038 _ _ _] -> [_ _ _ _ _ w1073 _]
              seq-local: [_ _ _ _ w1051 _ _] -> [_ _ _ _ _ w1071 _]
              seq-local: [_ w1006 _ _ _ _ _] -> [_ _ _ _ _ _ w1084]
              seq-local: [_ _ w1032 _ _ _ _] -> [_ _ _ _ _ w1070 _]
              tunnel: w1000 -> [_ w1008 _ _ _ _ _]
              frame #0 {
                n569 = Build Array("Name", "Channel", "High limit", "Low limit") -> (w1001:string[])
              }
              frame #1 {
                n570 = global read "Meas_global.vi" "LDA data"() -> (w1006:enum16{"No LDA data", "Take LDA data"})
                n571 = case shown="\"Take LDA data\"" w1006 {
                  tunnel: w1008 -> [_ w1019]
                  tunnel: [string[][] [] w1016] -> w1007
                  frame "No LDA data" {
                  }
                  frame "Take LDA data" {
                    n572 = global read "LDA_meas_global_1.vi" "Max Vel BSA1"() -> (w1011:dbl)
                    n573 = global read "LDA_meas_global_1.vi" "Min Vel BSA1"() -> (w1010:dbl)
                    n574 = global read "LDA_meas_global_1.vi" "Vel Comp BSA1"() -> (w1020:string)
                    n575 = case shown="\"2D\"" w1019 {
                      tunnel: [string[] [] w1025] -> w1017
                      frame "1D" {
                      }
                      frame "2D" {
                        n576 = global read "LDA_meas_global_2.vi" "Max Vel BSA2"() -> (w1024:dbl)
                        n577 = global read "LDA_meas_global_2.vi" "Min Vel BSA2"() -> (w1023:dbl)
                        n578 = global read "LDA_meas_global_2.vi" "Vel Comp BSA2"() -> (w1026:string)
                        n579 = Format Into String(format string="%.1f m/s" ("Format String"), w1023) -> (resulting string=w1031:string)  [unwired: 2 in, 1 out]
                        n580 = Format Into String(format string="%.1f m/s" ("Format String"), w1024) -> (resulting string=w1030:string)  [unwired: 2 in, 1 out]
                        n581 = Build Array("LDA", w1026, w1030, w1031) -> (w1025:string[])
                      }
                    }
                    n582 = Format Into String(format string="%.1f m/s" ("Format String"), w1010) -> (resulting string=w1012:string)  [unwired: 2 in, 1 out]
                    n583 = Format Into String(format string="%.1f m/s" ("Format String"), w1011) -> (resulting string=w1013:string)  [unwired: 2 in, 1 out]
                    n584 = Build Array("LDA", w1020, w1013, w1012) -> (w1018:string[])
                    n585 = Build Array(w1018, w1017) -> (w1016:string[][])
                  }
                }
              }
              frame #2 {
                n586 = global read "Meas_global.vi" "PWA Data"() -> (w1033:T31)
                n587 = case shown="\"One Ch PWA\"" w1033 {
                  tunnel: [string[][] [] w1035] -> w1032
                  frame "No PWA Data" {
                  }
                  frame "One Ch PWA" {
                    n588 = Build Array("PWA") -> (w1036:string[])
                    n589 = Build Array(w1036) -> (w1035:string[][])
                  }
                }
              }
              frame #3 {
                n590 = global read "Meas_global.vi" "Ch & spans"() -> (w1039:T28[])
                n591 = for {
                  tunnel: w1039 -> [w1050] mode=indexing
                  tunnel: [w1046] -> w1038 mode=indexing
                  n592 = Unbundle By Name(w1050) -> ("Var name"=w1049:string, "Ch No"=w1048:i16, "high limit (10V)"=w1043:sgl, "low limit (-10V)"=w1042:sgl)
                  n593 = Format Into String(format string="%.1f Volts" ("Format String"), w1043) -> (resulting string=w1041:string)  [unwired: 2 in, 1 out]
                  n594 = Format Into String(format string="%.1f Volts" ("Format String"), w1042) -> (resulting string=w1040:string)  [unwired: 2 in, 1 out]
                  n595 = Number To Decimal String(number=w1048) -> (decimal integer string=w1047:string)  [unwired: 1 out]
                  n596 = Build Array(w1049, w1047, w1041, w1040) -> (w1046:string[])
                }
              }
              frame #4 {
                n597 = global read "Meas_global.vi" "Analysis Info cluster"() -> (w1059:T22[])
                n598 = for {
                  tunnel: w1059 -> [w1069] mode=indexing
                  tunnel: [w1068] -> w1057 mode=indexing
                  n599 = Unbundle By Name(w1069) -> ("Inst name"=w1068:string)
                }
                n600 = global read "Meas_global.vi" "correlate"() -> (w1058:i32[][])
                n601 = for {
                  tunnel: w1058 -> [w1064] mode=indexing
                  tunnel: w1057 -> [w1063]
                  tunnel: "Correlating" -> [w1062]
                  tunnel: [w1060] -> w1052 mode=indexing
                  n602 = for {
                    tunnel: w1064 -> [w1067] mode=indexing
                    tunnel: w1063 -> [w1066]
                    tunnel: [w1065] -> w1061 mode=indexing
                    n603 = Index Array(array=w1066, index=w1067) -> (element=w1065:string)
                  }
                  n604 = Build Array (concatenate)(w1062, w1061) -> (w1060:string[])
                }
                n605 = Initialize Array("", 5 ("Dimension Size")) -> (w1053:string[])
                n606 = Build Array (concatenate)(w1053, w1052) -> (w1051:string[][])
              }
              frame #5 {
                n607 = Build Array (concatenate)(w1075, w1074, w1070, w1073, w1071) -> (w1072:string[][])
                n608 = local write "Statistics"(w1072) -> ()
              }
              frame #6 {
                n609 = case shown="\"Take LDA data\"" w1084 {
                  tunnel: [string[] [] w1086] -> w1081
                  frame "No LDA data" {
                  }
                  frame "Take LDA data" {
                    n610 = global read "Meas_global.vi" "Synchronise with LDA"() -> (w1091:bool)
                    n611 = global read "Meas_global.vi" "Ch & spans"() -> (w1094:T28[])
                    n612 = Array Size(array=w1094) -> (size(s)=w1093:i32)
                    n613 = Greater Than 0?(x=w1093) -> (x > 0?=w1092:bool)
                    n614 = Compound Arithmetic op=AND(w1091, w1092) -> (w1090:bool)
                    n615 = Select(t="Synchronised with LDA", s=w1090, f="") -> (s? t:f=w1087:string)
                    n616 = Build Array(w1087) -> (w1086:string[])
                  }
                }
                n617 = global read "Meas_global.vi" "Continuous time trace?"() -> (w1076:bool)
                n618 = Select(t="Continuous Time Trace", s=w1076, f="") -> (s? t:f=w1080:string)
                n619 = Build Array (concatenate)(w1081, w1080) -> (w1079:string[])
                n620 = Build Array(w1079) -> (w1078:string[][])
                n621 = Transpose 2D Array(2D array=w1078) -> (transposed array=w1077:string[][])
                n622 = local write "Diagnostic info"(w1077) -> ()
              }
            }
          }
        }
      }
      frame #19 {
        n623 = local read "File"() -> (w1105:T5)
        n624 = Equal?(x=Setup."Run Program" ("setup"), y=w1106) -> (x = y?=w1103:bool)
        n625 = Not Equal?(x=w1105, y=Save_Data."Save No Data" ("File")) -> (x != y?=w1104:bool)
        n626 = global read "Meas_global.vi" "Repeat Measurement?"() -> (w1095:bool)
        n627 = Compound Arithmetic op=AND(invert w1095, w1103, w1104) -> (w1102:bool)
        n628 = Get Date/Time In Seconds() -> (seconds since 1Jan1904=w1099:timestamp)
        n629 = To Double Precision Float(number=w1099) -> (double precision float=w1097:dbl)
        n630 = local read "Setup filename"() -> (w1100:string)
        n631 = case shown="False" w1102 {
          tunnel: w1105 -> [_ _]
          tunnel: w1097 -> [w1109 w1142]
          tunnel: w1100 -> [w1108 w1141]
          tunnel: w1096 -> [w1107 w1140]
          frame True {
            n632 = stacked-sequence {
              seq-local: [_ w1113 _] -> [_ _ w1133]
              tunnel: w1109 -> [w1112 _ _]
              tunnel: w1108 -> [w1111 _ _]
              tunnel: w1107 -> [w1110 _ _]
              frame #0 {
                n633 = call "Write_Results_file.vi"("Experiment start time"=w1110, "Experiment End time"=w1112, "Setup filename"=w1111) -> ()  [unwired: 4 out]
              }
              frame #1 {
                w1118 = FALSE  # Empty list
                n634 = global read "Meas_global.vi" "Raw data file"() -> (w1117:path)
                n635 = global read "Trav_pos_global.vi" "Top level setup filename"() -> (w1115:path)
                n636 = global read "Meas_global.vi" "Start Time of experiment"() -> (w1114:dbl)
                n637 = Strip Path(path=w1117) -> (stripped path=w1113:path)  [unwired: 1 out]
                n638 = Empty String/Path?(string/path=w1115) -> (empty?=w1116:bool)
                n639 = case shown="False" w1116 {
                  tunnel: w1115 -> [w1132 _]
                  tunnel: w1113 -> [w1130 _]
                  tunnel: w1114 -> [w1128 _]
                  frame False {
                    n640 = call "Sec_to_date_filename.vi"("seconds"=w1128) -> ("Day"=w1127:string, "Time"=w1126:string)  [unwired: 2 out]
                    n641 = Format Into String(format string="Cmd_%s_%s.xls", w1127, w1126) -> (resulting string=w1124:string)  [unwired: 2 in, 1 out]
                    n642 = call "Fast_string_Replace.vi"("Replace match with:"="-", "Input String"=w1124, "regular expression"=":") -> ("Output String"=w1121:string)  [unwired: 2 out]
                    n643 = call "Fast_string_Replace.vi"("Replace match with:"="", "Input String"=w1121, "regular expression"=" ") -> ("Output String"=w1119:string)  [unwired: 2 out]
                    n644 = Build Path(base path=w1130, name or relative path=w1119) -> (appended path=w1129:path)
                    n645 = Copy(10:w1129, 11:w1132) -> ()  [unwired: 1 in, 5 out]
                  }
                  frame True {
                  }
                }
                n646 = call "Remember_RD_Folders.vi"("Empty list"=w1118, "Folders to Remember"=w1113) -> ()  [unwired: 1 out]
              }
              frame #2 {
                n647 = global read "Meas_global.vi" "LDA data"() -> (w1134:enum16{"No LDA data", "Take LDA data"})
                n648 = case shown="\"Take LDA data\"" w1134 {
                  tunnel: w1133 -> [_ w1138]
                  frame "No LDA data" {
                  }
                  frame "Take LDA data" {
                    w1136 = "LDA_Probe_Orientation.txt" ("name or relative path")
                    n649 = call "Setup_Filepath.vi"("Setup File Type"=Setup_Filetype."General", "Filename in"=w1136) -> ("Filename Out"=w1135:path)  [unwired: 1 out]
                    n650 = Build Path(base path=w1138, name or relative path=w1136) -> (appended path=w1139:path)
                    n651 = Copy(10:w1139, 11:w1135) -> ()  [unwired: 1 in, 5 out]
                  }
                }
              }
            }
          }
          frame False {
            n652 = global read "Meas_global.vi" "Raw data option"() -> (w1143:enum16{"Save raw data", "Raw data not saved"})
            n653 = case shown="\"Save raw data\"" w1143 {
              tunnel: w1140 -> [w1146 _]
              tunnel: w1142 -> [w1145 _]
              tunnel: w1141 -> [w1144 _]
              frame "Save raw data" {
                n654 = stacked-sequence {
                  tunnel: w1146 -> [_ w1155]
                  tunnel: w1145 -> [_ w1154]
                  tunnel: w1144 -> [_ w1152]
                  frame #0 {
                    n655 = global read "Meas_global.vi" "Current Block No"() -> (w1147:i32)
                    n656 = global write "Meas_global.vi" "Requested No of blocks"(w1147) -> ()
                  }
                  frame #1 {
                    n657 = call "Create_Raw_data_file.vi"("No of averages"=1, "End time"=w1154, "Start time"=w1155, "Setup filename"=w1152) -> ("Values"=w1150:string[][], "Column headers"=w1151:string[])  [unwired: 2 out]
                    n658 = Index Array(array=w1150, index (row)=0) -> (element=w1148:string[])  [unwired: 1 in]
                    n659 = global write "Dynamic_call_global.ph.vi" "Plug in values"(w1148) -> ()
                    n660 = global write "Dynamic_call_global.ph.vi" "Plug in titles"(w1151) -> ()
                  }
                }
              }
              frame "Raw data not saved" {
              }
            }
          }
        }
      }
      frame #20 {
        n661 = stacked-sequence {
          seq-local: [w1169 _ _] -> [_ w1176 _]
          seq-local: [w1166 _ _] -> [_ w1175 w1215]
          seq-local: [w1161 _ _] -> [_ _ w1216]
          tunnel: w1157 -> [w1174 _ _]
          tunnel: w1156 -> [w1159 _ _]
          frame #0 {
            n662 = global read "Meas_global.vi" "Raw data file"() -> (w1167:path)
            n663 = global read "Meas_global.vi" "Raw data option"() -> (w1173:enum16{"Save raw data", "Raw data not saved"})
            n664 = Equal?(x=Setup."Run Program" ("setup"), y=w1174) -> (x = y?=w1164:bool)
            n665 = Strip Path(path=w1167) -> (stripped path=w1162:path)  [unwired: 1 out]
            n666 = global read "Extra_Commands_Global.vi" "Add Height to Local Floor Height"() -> (w1160:string)
            n667 = Equal?(x=w1173, y=enum16{"Save raw data", "Raw data not saved"}."Save raw data" ("Raw data option")) -> (x = y?=w1163:bool)
            n668 = call "Extra_Commands.vi"("String to Search"=w1159, "Command"=w1160) -> ("Command Found"=w1158:bool)  [unwired: 1 in, 4 out]
            n669 = Build Path(base path=w1162, name or relative path="VI_History.xls") -> (appended path=w1166:path)
            n670 = Compound Arithmetic op=AND(w1164, w1163, w1158) -> (w1161:bool)
            n671 = call "Does_file_exist_(simple).vi"("Pathname"=w1166) -> ("exists?"=w1171:bool)
            n672 = Not(x=w1171) -> (.not. x?=w1170:bool)
            n673 = Compound Arithmetic op=AND(w1170, w1164, w1163) -> (w1169:bool)
          }
          frame #1 {
            n674 = case shown="True" w1176 {
              tunnel: w1175 -> [_ w1177]
              frame False {
              }
              frame True {
                n675 = stacked-sequence {
                  tunnel: w1177 -> [w1183 w1191]
                  frame #0 {
                    w1180 = FALSE  # Lock File
                    n676 = global read "Meas_global.vi" "ProgRevisionInfo"() -> (w1179:string)
                    n677 = call "Characters_to_string.vi"("Characters to write"=w1179, "Label for characters"="Prog Revision info") -> ("Output string"=w1185:string)
                    n678 = call "Date_and_Time_to_string.vi"() -> ("Date and time (spreadsheet)"=w1186:string)
                    n679 = call "Get_mod_dates.vi"() -> ("error out"=w1184:errorcluster, "Output string"=w1181:string)  [unwired: 1 in, 3 out]
                    n680 = call "EnFlo_Error_Handler.vi"("error in (no error)"=w1184) -> ()  [unwired: 2 in, 3 out]
                    n681 = Concatenate Strings(w1186, w1185, w1181) -> (w1182:string)
                    n682 = call "Write_Characters_To_File.vi"("file path (dialog if empty)"=w1183, "character string"=w1182, "Lock File"=w1180) -> ()  [unwired: 2 in, 4 out]
                  }
                  frame #1 {
                    n683 = global read "Trav_pos_global.vi" "Traverses to Move"() -> (w1189:string[])
                    n684 = global read "Constants_global.vi" "Traverse folder"() -> (w1190:path)
                    n685 = Strip Path(path=w1191) -> (stripped path=w1188:path)  [unwired: 1 out]
                    n686 = for {
                      tunnel: w1190 -> [w1203]
                      tunnel: w1189 -> [w1199] mode=indexing
                      tunnel: w1188 -> [w1200]
                      tunnel: string[] ["Traverse_Preferences.txt", "Traverse_Setup.xls"] ("Traverses to Move") -> [w1192]
                      n687 = Build Path(base path=w1203, name or relative path=w1199) -> (appended path=w1195:path)
                      n688 = Build Path(base path=w1195, name or relative path="Trav_Space_Files" ("Substring")) -> (appended path=w1202:path)
                      n689 = Build Path(base path=w1202, name or relative path="Selected_Filename.txt" ("Substring")) -> (appended path=w1207:path)
                      n690 = call "Create_directory_path.vi"("Path name"=w1207) -> ("Path name Out"=w1206:path)  [unwired: 1 in, 1 out]
                      n691 = Build Path(base path=w1200, name or relative path=w1199) -> (appended path=w1194:path)
                      n692 = for {
                        tunnel: w1195 -> [w1214]
                        tunnel: w1194 -> [w1212]
                        tunnel: w1192 -> [w1210] mode=indexing
                        n693 = Build Path(base path=w1214, name or relative path=w1210) -> (appended path=w1213:path)
                        n694 = Build Path(base path=w1212, name or relative path=w1210) -> (appended path=w1209:path)
                        n695 = call "Create_directory_path.vi"("Path name"=w1209) -> ("Path name Out"=w1208:path)  [unwired: 1 in, 1 out]
                        n696 = Copy(9:TRUE ("overwrite (F)"), 10:w1208, 11:w1213) -> ()  [unwired: 2 in, 3 out]
                      }
                      n697 = call "Read_File_Simple.vi"("Filename"=w1206) -> ("string"=w1197:string)  [unwired: 2 in, 7 out]
                      n698 = Build Path(base path=w1194, name or relative path=w1197) -> (appended path=w1198:path)
                      n699 = Build Path(base path=w1202, name or relative path=w1197) -> (appended path=w1201:path)
                      n700 = call "Create_directory_path.vi"("Path name"=w1198) -> ("Path name Out"=w1196:path)  [unwired: 1 in, 1 out]
                      n701 = Copy(9:TRUE ("overwrite (F)"), 10:w1196, 11:w1201) -> ()  [unwired: 2 in, 3 out]
                    }
                  }
                }
              }
            }
          }
          frame #2 {
            n702 = case shown="True" w1216 {
              tunnel: w1215 -> [_ w1231]
              frame False {
              }
              frame True {
                n703 = global read "Meas_global.vi" "Start Time of experiment"() -> (w1220:dbl)
                n704 = Strip Path(path=w1231) -> (stripped path=w1230:path)  [unwired: 1 out]
                n705 = call "Sec_to_date_filename.vi"("seconds"=w1220) -> ("Day"=w1228:string, "Time"=w1227:string)  [unwired: 2 out]
                n706 = Format Into String(format string="Floor_Surface_%s_%s.xls", w1228, w1227) -> (resulting string=w1225:string)  [unwired: 2 in, 1 out]
                n707 = call "Fast_string_Replace.vi"("Replace match with:"="-", "Input String"=w1225, "regular expression"=":") -> ("Output String"=w1222:string)  [unwired: 2 out]
                n708 = call "Fast_string_Replace.vi"("Replace match with:"="", "Input String"=w1222, "regular expression"=" ") -> ("Output String"=w1219:string)  [unwired: 2 out]
                n709 = Build Path(base path=w1230, name or relative path=w1219) -> (appended path=w1218:path)
                n710 = call "Does_file_exist_(simple).vi"("Pathname"=w1218) -> ("exists?"=w1217:bool)
                n711 = case shown="False" w1217 {
                  tunnel: w1218 -> [w1232 _]
                  frame False {
                    n712 = call "Setup_Filepath.vi"("Setup File Type"=Setup_Filetype."General", "Filename in"="Floor_Surface_Mapping.xls") -> ("Filename Out"=w1234:path)  [unwired: 1 out]
                    n713 = Copy(9:TRUE ("overwrite (F)"), 10:w1232, 11:w1234) -> ()  [unwired: 2 in, 3 out]
                  }
                  frame True {
                  }
                }
              }
            }
          }
        }
      }
      frame #21 {
        n714 = local read "Correlate?"() -> (w1241:T9)
        n715 = case shown="\"Run Program\"" w1238 {
          tunnel: w1238 -> [w1243 _ _ _]
          tunnel: [w1243 w1256 w1257 w1258] -> w1237
          frame "Run Program" {
            n716 = global read "Meas_global.vi" "Analysis Info cluster"() -> (w1242:T22[])
            n717 = for {
              tunnel: w1242 -> [w1254] mode=indexing
              stop <- w1244 stop-if-true
              w1251 = "Pitot ("
              n718 = Unbundle By Name(w1254) -> ("U"=w1245:dbl, "Inst name"=w1250:string)
              n719 = String Length(string=w1251) -> (length=w1253:i32)
              n720 = String Subset(string=w1250, length (rest)=w1253) -> (substring=w1252:string)  [unwired: 1 out]
              n721 = Equal?(x=w1252, y=w1251) -> (x = y?=w1247:bool)
              n722 = call "Match_Pat_Case_In.vi"("String to match"="ref", "String"=w1250) -> ("offset past match"=w1248:i32)  [unwired: 1 in, 3 out]
              n723 = Greater Or Equal To 0?(x=w1248) -> (x >= 0?=w1246:bool)
              n724 = And(x=w1246, y=w1247) -> (x .and. y?=w1244:bool)
              n725 = case shown="True" w1244 {
                tunnel: w1245 -> [_ w1255]
                frame False {
                }
                frame True {
                  n726 = call "Log_Reference_Velocity.vi"("Measured Velocity"=w1255) -> ()  [unwired: 1 out]
                }
              }
            }
          }
          frame "Show Setup" {
            w1256 = Setup."Run Program"  # setup
          }
          frame "Save Current Setup" {
            w1257 = Setup."Run Program"  # setup
          }
          frame "Setup Front Panel" {
            w1258 = Setup."Run Program"  # setup
          }
        }
        n727 = case shown="\"Show correlation panel\"" w1241 {
          tunnel: [T9."Cross correlation off" T9."Correlate without activating panel" T9."Correlate without activating panel"] -> w1240
          frame "Cross correlation off" {
          }
          frame "Show correlation panel" {
          }
          frame "Correlate without activating panel" {
          }
        }
        n728 = local write "Correlate?"(w1240) -> ()
        n729 = global write "Meas_global.vi" "Remote control"(FALSE ("Remote control")) -> ()
        n730 = call "Program_Active.vi"() -> ()  [unwired: 1 in]
        n731 = local write "setup"(w1237) -> ()
      }
      frame #22 {
        w1267 = FALSE  # Dialog Box (T)
        n732 = global read "Meas_global.vi" "Post Process"() -> (w1262:T2)
        n733 = case shown="\"Take New Data\"" w1262 {
          frame "Take New Data" {
            n734 = global read "Meas_global.vi" "Requested Sampling rate"() -> (w1290:dbl)
            n735 = global read "Meas_global.vi" "Analysis Info cluster"() -> (w1286:T22[])
            n736 = Divide(x=w1290, y=10.0) -> (x/y=w1287:dbl)
            n737 = Max & Min(x=w1287, y=100.0) -> (min(x,y)=w1285:dbl)  [unwired: 1 out]
            n738 = for {
              tunnel: w1286 -> [w1321] mode=indexing
              tunnel: w1285 -> [w1316]
              tunnel: [w1314] -> w1282 mode=indexing if=w1310
              tunnel: [w1311] -> w1273 mode=indexing if=w1312
              tunnel: [w1311] -> w1271 mode=indexing if=w1310
              n739 = Unbundle By Name(w1321) -> ("Inst name"=w1315:string, "Av Sampling Rate"=w1314:dbl, "Inst type"=w1320:T14)
              n740 = Equal?(x=w1320, y=Inst_type."LDA Vel" ("Inst type")) -> (x = y?=w1310:bool)
              n741 = Greater Than 0?(x=w1314) -> (x > 0?=w1317:bool)
              n742 = Less?(x=w1314, y=w1316) -> (x < y?=w1318:bool)
              n743 = Compound Arithmetic op=AND(w1318, w1317, w1310) -> (w1312:bool)
              n744 = Format Into String(format string="The %s currently has a data rate of %d Hz\n", w1315, w1314) -> (resulting string=w1311:string)  [unwired: 2 in, 1 out]
            }
            n745 = Array Max & Min(array=w1282) -> (max value=w1280:dbl, min value=w1279:dbl)  [unwired: 2 out]
            n746 = Array Size(array=w1282) -> (size(s)=w1281:i32)
            n747 = Concatenate Strings(w1271) -> (w1270:string)
            n748 = Concatenate Strings(w1273) -> (w1272:string)
            n749 = Empty String/Path?(string/path=w1272) -> (empty?=w1284:bool)
            n750 = case shown="False" w1284 {
              tunnel: [w1301 FALSE] -> w1283
              frame False {
                n751 = global read "Preference_global.vi" "Rig Setup"() -> (w1307:string)
                n752 = Concatenate Strings("Status:of:", w1307) -> (w1306:string)
                n753 = Build Array(w1306) -> (w1305:string[])
                n754 = call "Get_Current_Scan_client.vi"("ADAM Ch Names"=w1305) -> ("Numerical Values"=w1304:dbl[])  [unwired: 1 in, 2 out]
                n755 = Index Array(array=w1304) -> (element=w1303:dbl)  [unwired: 1 in]
                n756 = Equal?(x=2.0, y=w1303) -> (x = y?=w1301:bool)
              }
              frame True {
              }
            }
            n757 = case shown="True" w1283 {
              tunnel: w1272 -> [_ w1296]
              frame False {
              }
              frame True {
                w1299 = FALSE  # Dialog Box (T)
                n758 = Bundle By Name(cluster=errorcluster {"status"=TRUE, "code"=0, "source"=""} ("error in (no error)"), "source"=w1296) -> (w1298:errorcluster)
                n759 = call "EnFlo_Error_Handler.vi"("error in (no error)"=w1298, "Error Type"="Low LDA Sampling Rate", "Dialog Box (T)"=w1299) -> ()  [unwired: 3 out]
              }
            }
            n760 = Greater Than 0?(x=w1281) -> (x > 0?=w1276:bool)
            n761 = Divide(x=w1280, y=w1279) -> (x/y=w1274:dbl)
            n762 = Greater?(x=w1274, y=4.0) -> (0:w1277:bool)
            n763 = And(x=w1276, y=w1277) -> (x .and. y?=w1275:bool)
            n764 = case shown="True" w1275 {
              tunnel: w1270 -> [_ w1291]
              frame False {
              }
              frame True {
                w1294 = FALSE  # Dialog Box (T)
                n765 = Bundle By Name(cluster=errorcluster {"status"=TRUE, "code"=0, "source"=""} ("error in (no error)"), "source"=w1291) -> (w1293:errorcluster)
                n766 = call "EnFlo_Error_Handler.vi"("error in (no error)"=w1293, "Error Type"="LDA Data rate ratio greater than 4", "Dialog Box (T)"=w1294) -> ()  [unwired: 3 out]
              }
            }
          }
          frame "Post Process Raw Data File" {
          }
        }
        n767 = global read "Meas_global.vi" "Over/Under string"() -> (w1265:string)
        n768 = Empty String/Path?(string/path=w1265) -> (empty?=w1264:bool)
        n769 = Not(x=w1264) -> (.not. x?=w1263:bool)
        n770 = Bundle By Name(cluster=errorcluster {"status"=FALSE, "code"=0, "source"=""} ("error in (no error)"), "source"=w1265, "status"=w1263) -> (w1268:errorcluster)
        n771 = call "EnFlo_Error_Handler.vi"("error in (no error)"=w1268, "Error Type"="Signal Clipping", "Dialog Box (T)"=w1267) -> ()  [unwired: 3 out]
      }
      frame #23 {
        w1324 = string[] [] ("Per Block Plug Ins Extra")
        n772 = Empty String/Path?(string/path=w1328) -> (empty?=w1327:bool)
        n773 = global read "Dynamic_call_global.ph.vi" "Final Plug Ins"() -> (w1329:string[])
        n774 = case shown="True" w1327 {
          tunnel: w1328 -> [w1340 _]
          frame False {
            n775 = local read "Comments"() -> (w1339:string)
            n776 = call "Fast_string_Replace.vi"("Replace match with:"="", "Input String"=w1339, "regular expression"=w1340) -> ("Output String"=w1338:string)  [unwired: 2 out]
            n777 = local write "Comments"(w1338) -> ()
          }
          frame True {
          }
        }
        n778 = call "Plug_in_Directories.vi"() -> ("Final"=w1325:path)  [unwired: 3 out]
        n779 = for {
          tunnel: w1329 -> [w1343] mode=indexing
          tunnel: w1325 -> [w1342]
          w1346 = FALSE  # Dialog Box (T)
          n780 = Build Path(base path=w1342, name or relative path=w1343) -> (appended path=w1341:path)
          n781 = global read "Dynamic_call_global.ph.vi" "Plug in"() -> (w1351:refnum<vi>)
          n782 = Open VI Reference(type specifier VI Refnum (for type only)=w1351, vi path=w1341) -> (vi reference=w1350:refnum<vi>, error out=w1349:errorcluster)  [unwired: 2 in, 2 out]
          n783 = call-by-ref "?"(reference=w1350, error in=w1349) -> (reference out=w1347:refnum<vi>, error out=w1348:errorcluster)  [unwired: 6 in, 2 out]
          n784 = Close Reference(reference=w1347, error in (no error)=w1348) -> (error out=w1344:errorcluster)
          n785 = call "EnFlo_Error_Handler.vi"("error in (no error)"=w1344, "Error Type"="Running Final Plug In", "Dialog Box (T)"=w1346) -> ()  [unwired: 3 out]
        }
        n786 = global read "Meas_global.vi" "Repeat Measurement?"() -> (w1326:bool)
        n787 = case shown="True" w1326 {
          tunnel: w1323 -> [_ w1336]
          tunnel: [FALSE w1331] -> w1322
          frame False {
          }
          frame True {
            n788 = global read "Meas_global.vi" "Post Process"() -> (w1334:T2)
            n789 = Equal To 0?(x=w1336) -> (x = 0?=w1332:bool)
            n790 = Equal?(x=w1334, y=Post_Process."Post Process Raw Data File" ("Post Process")) -> (x = y?=w1333:bool)
            n791 = And(x=w1333, y=w1332) -> (x .and. y?=w1331:bool)
          }
        }
        n792 = global write "Dynamic_call_global.ph.vi" "Per Block Plug Ins Extra"(w1324) -> ()
        n793 = global write "Dynamic_call_global.ph.vi" "Initial Plug Ins Extra"(w1324) -> ()
      }
      frame #24 {
        n794 = global read "Meas_global.vi" "Post Process"() -> (w1358:T2)
        n795 = local read "stop"() -> (w1364:bool)
        n796 = Equal?(x=w1359, y=Setup."Run Program" ("setup")) -> (x = y?=w1355:bool)
        n797 = Equal?(x=w1358, y=Post_Process."Take New Data" ("Post Process")) -> (x = y?=w1356:bool)
        n798 = And(x=w1355, y=w1356) -> (x .and. y?=w1354:bool)
        n799 = case shown="False" w1364 {
          tunnel: [Multi_Run_Status."Continue" ("Status Out") Multi_Run_Status."Terminate Run" ("Status Out")] -> w1362
          frame False {
          }
          frame True {
            n800 = local write "stop"(FALSE) -> ()
          }
        }
        n801 = case shown="True" w1354 {
          tunnel: w1362 -> [w1365 w1368]
          tunnel: [w1365 w1370] -> w1361
          frame False {
          }
          frame True {
            n802 = local read "Raw data file"() -> (w1369:path)
            n803 = Path to Array of Strings(0:w1369) -> (2:w1371:string[])  [unwired: 1 out]
            n804 = Index Array(array=w1371, index=0 ("Index")) -> (element=w1367:string)
            n805 = Build Array(w1367) -> (w1366:string[])
            n806 = for {
              tunnel: w1366 -> [w1375] mode=indexing
              shift-right: [w1373] -> w1370
              shift-left: w1368 -> [w1374]
              n807 = call "Warn_on_low_HD_space.vi"("Status In"=w1374, "HD name"=w1375) -> ("Status Out"=w1373:T1)  [unwired: 6 out]
            }
          }
        }
        "Status Out" <- w1361
        n808 = global write "Trav_pos_global.vi" "Dummy Measurement?"(FALSE ("Dummy Measurement?")) -> ()
        n809 = global write "Plug_in_data_global.vi" "Server Channels to log"(string[] [] ("Server Channels to log")) -> ()
        n810 = global write "Meas_global.vi" "Extra Comments"("") -> ()
      }
    }
  }
